vi "main 0.9.0.vi"() -> ()   [LabVIEW 2020]
uses:
  subvi/Newport ESP301/Newport ESP301.lvlib
  subvi/sp_manip.llb/sp_manip_lib.lvlib
  subvi/sp_manip.llb/tcp_gateway.lvlib
  subvi/PHOIBOS/DEFINITIONS/DEF_dev_type.ctl
  subvi/PHOIBOS/DEFINITIONS/DEF_dev_state.ctl
  <vilib>/Utility/file.llb/Write Delimited Spreadsheet (DBL).vi
panel:
  in  "BasePath":path=path "C:/Users/femtolab_admin/Desktop"
  in  "cam_liveavg":bool caption="live average"
  out "G2":dbl[](graph)=[263.145, 1605.73, 2749.3099999999995, 2478.555, 1442.25, 1948.3050000000003, 3089.7200000000003, 2536.98, 1326.19, 1765.79, 1232.225, 654.385, 1490.405, 2145.9949999999994, 2745.5350000000003, 2855.805, 2377.34, 3038.8550000000005, 2930.365, 1581.4399999999998, 1915.805, 2285.69, 1454.7, 796.3300000000002, 1536.01, 2295.5749999999994, 2779.0199999999995, 3696.9249999999997, 2846.545, 1289.3599999999997, 1847.72, 1825.405, 803.2200000000001, 899.645, 662.7249999999999, 467.48, 1104.215, 1475.7500000000002, 1531.1799999999996, 1721.645, 2162.135, 2133.0849999999996, 1255.03, 851.9999999999999, 1367.655, 1933.275, 1143.7749999999999, 741.21, 1149.32, 1642.1000000000001, 1020.995, 530.395, 1069.84, 1391.8100000000002, 1042.03, 1818.6999999999998, 4069.855, 5797.8550000000005, 5827.435, 5055.504999999999, 2832.8900000000003, 1841.045, 2277.75, 1826.1050000000002, 1200.9950000000001, 1153.9649999999997, 1637.5700000000002, 1942.64, 2197.6200000000003, 2863.3550000000005, 3618.209999999999, 3665.4650000000006, 2446.0150000000003, 1297.435, 1719.3950000000002, 2087.6949999999997, 1830.3849999999998, 2194.1750000000006, 2078.385, 1316.6150000000002, 1545.65, 2258.02, 2764.9700000000003, 3237.4200000000005, 1775.6750000000002, 414.32499999999993, 416.3499999999999, 394.96999999999997, 916.545, 1994.625, 3344.8700000000003, 3847.5449999999996, 2925.8199999999997, 2678.08, 2296.67, 1098.0200000000002, 1790.3249999999998, 3163.6549999999997, 3836.945, 3560.370000000001, 2904.32, 2978.2800000000007, 2652.4350000000004, 1855.06, 1771.505, 2235.425, 2266.66, 1323.0649999999998, 1657.0400000000004, 2715.995, 2765.325, 3528.2700000000004, 3528.8050000000003, 2683.3199999999997, 2324.45, 3198.8550000000005, 3244.14, 2267.045, 2132.2949999999996, 2030.79, 907.7950000000001, 1260.255, 1373.4299999999998, 1413.51, 1800.5400000000004, 1761.2450000000003, 1803.33, 2071.47, 2702.28, 3012.6950000000006, 3130.8699999999994, 3128.955, 3589.63, 2744.915000000001, 2048.795, 1583.935, 1144.4499999999998, 1851.075, 1980.545, 1512.4350000000002, 581.935, 731.1850000000001, 621.78, 164.225, 0.0, 0.0, 0.0, 0.0, 0.0, 0.0, 0.0, 0.0, 0.0, 0.0, 0.0, 0.0, 0.0, 124.49000000000001, 496.75, 551.67, 103.64, 0.0, 0.0, 0.0, 0.0, 54.11, 80.15, 0.0, 0.0, 0.0, 0.0, 0.0, 0.0, 0.0, 0.0, 0.0, 0.0, 0.0, 0.0, 0.0, 51.42, 410.03499999999997, 580.33, 174.89999999999998, 0.0, 0.0, 0.0, 0.0, 0.0, 0.0, 0.0, 0.0, 0.0, 0.0, 0.0, 0.0, 0.0, 0.0, 0.0, 0.0, 0.0, 0.0, 0.0, 0.0, 0.0, 0.0, 0.0, 0.0, 0.0, 0.0, 0.0, 0.0, 0.0, 0.0, 0.0, 0.0, 0.0, 0.0, 0.0, 0.0, 0.0, 0.0, 0.0, 0.0, 0.0, 490.6700000000001, 1051.7849999999999, 758.91, 53.42, 0.0, 0.0, 0.0, 60.32, 125.305, 0.0, 0.0, 121.69999999999999, 0.0, 0.0, 0.0, 184.825, 263.615, 0.0, 0.0, 0.0, 0.0, 0.0, 389.45000000000005, 1030.345, 1047.415, 81.37, 0.0, 0.0, 0.0, 301.08, 452.075, 74.22, 0.0, 0.0, 0.0, 0.0, 0.0, 0.0, 0.0, 0.0, 139.67000000000002, 572.5749999999999, 971.985, 771.0349999999999, 693.04, 79.35499999999999, 0.0, 0.0, 0.0, 0.0, 0.0, 0.0, 0.0, 0.0, 0.0, 0.0, 0.0, 0.0, 0.0, 0.0, 0.0, 0.0, 0.0, 0.0, 0.0, 0.0, 0.0, 0.0, 0.0, 0.0, 0.0, 0.0, 0.0, 0.0, 0.0, 0.0, 0.0, 0.0, 0.0, 0.0, 0.0, 0.0, 0.0, 0.0, 0.0, 0.0, 0.0, 0.0, 0.0, 0.0, 0.0, 0.0, 0.0, 0.0, 0.0, 0.0, 0.0, 0.0, 0.0, 0.0, 0.0, 0.0, 0.0, 0.0, 0.0, 0.0, 0.0, 0.0, 0.0, 0.0, 0.0, 0.0, 0.0, 0.0, 0.0, 0.0, 0.0, 0.0, 0.0]
  out "cam_fps":dbl=19.771956531604918 caption="FPS" format="%.1g"
  out "sideimg":dbl[][](graph)
  in  "RunNumber":u16=3
  out "sum":dbl=307111.85500000004 format="%#.2g"
  out "max":dbl=632.85
  out "mainimg":dbl[][](graph)
  out "ESP_con?":bool=TRUE caption="ESP301"
  out "phoib_con?":bool caption="PHOIBOS"
  out "manip_con?":bool caption="manipulator"
  out "cam_con?":bool caption="camera"
  in  "main_close":bool
  in  "Tab Control":T1(tab)
  in  "manip_deltas":dbl[](array[numeric])=[0.0, 0.0, 0.0, 0.0, 10.0, 0.0] caption="delta" format="%#.5g"
  in  "aq.mode":enum32{"Radio Selection 1", "Radio Selection 2"}(radio)=enum."Radio Selection 2"
  out "snap_prog":dbl(slide)=1.0 scale=0.0..1.0
  in  "upper threshold":i32=15000
  in  "dark avg":i32=200
  in  "averages":i32=20 caption="N"
  in  "ESP_delta":dbl caption="relative [mm]"
  in  "ESP_-":bool
  in  "ESP_+":bool
  in  "ESP_go":bool
  in  "ESP_dest_t":dbl caption="[fs]"
  in  "ESP_dest":dbl=33.3075 caption="[mm]"
  in  "ESP_set_t0":bool
  in  "phoib_I_6s":dbl=3200.0
  in  "phoib_I_5s":dbl=1450.0
  in  "phoib_I_4s":dbl=4.558
  in  "phoib_I_3s":dbl=-7.0
  in  "phoib_I_2s":dbl=35.0
  in  "phoib_I_1s":dbl=21.9
  in  "phoib_standby":bool
  in  "phoib_set":bool
  out "phoib_I_6":dbl=3200.0 caption="Screen Voltage"
  out "phoib_I_5":dbl=1450.0 caption="Detctor Voltage"
  out "phoib_I_4":dbl=4.558 caption="Work Function"
  out "phoib_I_3":dbl=-7.0 caption="Coil Current"
  out "phoib_I_2":dbl=35.0 caption="Pass Energy"
  out "phoib_I_1":dbl=21.9 caption="Kinetic Energy"
  out "Saved Positions":string[][](table)=[["ertwertwert", "-2.299945", "-2.030214", "38.900024", "50.000762", "0.000887", "-97.998082"], ["uztgugt", "-14.999451", "-13.638894", "442.380066", "13.998380", "-1.893758", "-76.305838"], ["asdf", "-14.999451", "-13.638894", "442.380066", "13.998380", "-1.893758", "-76.305838"], ["test3", "-14.999451", "-13.638894", "441.380066", "13.998380", "-1.893758", "-76.305838"]]
  in  "Save Pos":bool
  in  "Load":bool
  in  "Delete":bool
  in  "ManipRel +":bool
  in  "ManipRel -":bool
  in  "Move Abs":bool
  in  "stop manip":bool
  in  "dest":dbl[](array[numeric])=[-2.6172862113166087, -0.009888298846365134, 68.5008544921875, -46.36280498847848, 1.1073518432055398, -218.56360350415366] caption="destination" format="%#.5g"
  out "axis":string[](array[string])=["x", "y", "z", "polar", "tilt", "azimut"]
  out "pos":dbl[](array[numeric])=[-2.6172862113166087, -0.009888298846365134, 68.5008544921875, -46.363686276590336, 11.108982061941884, -218.56360350415366] caption="position" format="%.5f"
  in  "Mode":T2(ring)=enum."WideAngleMode"
  in  "VoltageRange":enum16{"3.5kV", "1.5kV", "400V", "100V", "10V"}(ring)=enum."400V"
  out "ESP_pos":dbl=31.8299 caption="Position"
  out "ESP_delay":dbl=1000.0251574040519 caption="Delay"
  out "ESP_t0":dbl=31.68 caption="Time Zero @"
  out "phoib_I_7":dbl=-30.0 caption="Conversion Voltage"
  in  "phoib_I_7s":dbl=-30.0
  in  "phoib_I_8s":dbl=0.0039
  in  "phoib_I_9s":dbl=0.0039
  out "phoib_I_8":dbl=0.0039 caption="FD1"
  out "phoib_I_9":dbl=0.0039 caption="FD2"
  in  "gain":bool
  in  "exposure [ms]":u32=50
  in  "binning":u16(ring)=2 items=["X 1", "X 2", "X 4", "X 8"]
  in  "cam_dark?":bool=TRUE caption="subtract dark?"
  in  "cam_dark":bool
  in  "cam_saveimg":bool
  in  "e-size":u8
  in  "lower threshold":i32=50
  in  "count?":bool
  out "ETA":timestamp=timestamp(3543316529.918047 s since 1904-01-01) format="%<%H:%M:%S>T"
  in  "ROI Left":i32=1
  in  "ROI Right":i32=43
  in  "ROI Top":i32=2
  in  "ROI Bottom":i32=30
  out "moving?":bool[](array[boolean])
  in  "delscan_iters":u32=2 caption="iterations"
  out "scangraph":cluster{dbl[], dbl[]}(graph)={[-1000.0, -900.0, -800.0, -700.0, -600.0, -500.0, -400.0, -300.0, -200.0, -100.0, 0.0, 100.0, 200.0, 300.0, 400.0, 500.0, 600.0, 700.0, 800.0, 900.0, 1000.0], [2248493.455, 2199251.9574999977, 2219914.692499999, 2216051.6575000007, 2215958.2724999995, 2212331.0824999996, 2279964.2799999993, 2180338.027499999, 2266636.2549999994, 2285788.987499997, 2245434.3249999993, 2294344.6275000023, 2285044.407499997, 2174516.5600000033, 2247505.4800000004, 2255556.7350000003, 2175127.462499999, 2208174.432500001, 2235161.732500001, 2220116.9325000024, 2249237.3274999997, 0.0, 0.0, 0.0, 0.0, 0.0, 0.0, 0.0, 0.0, 0.0, 0.0, 0.0, 0.0, 0.0, 0.0, 0.0, 0.0, 0.0, 0.0, 0.0, 0.0, 0.0]}
  in  "delscan_abort":bool
  out "delscan_progress":u32(slide)=20 scale=0.0..21.0
  in  "delscan_go":bool
  out "delscan_pos":dbl=31.829896229 caption="current delay [fs]"
  in  "delscan_end":dbl=1000.0 caption="end [fs]"
  in  "delscan_stepsize":dbl=100.0 caption="stepsize [fs]"
  in  "delscan_start":dbl=-1000.0 caption="start [fs]"
  out "iteration":i32=2
  in  "manip_scan_steps":u32=3
  in  "Optimize":bool
  in  "manip_scan_delta":dbl[](array[numeric])=[0.0, 0.0, 0.0, 0.0, 1.0, 0.0] caption="delta" format="%#.5g"
  out "delscan_progress 2":u32(slide)=2 scale=0.0..3.0
  in  "abort":bool
  in  "manip_init":bool
  in  "manip_release":bool
  in  "phoib_init":bool
  in  "phoib_release":bool
  in  "ESP_init":bool
  in  "ESP_release":bool
  in  "ESP301 VISA":refnum<visa-resource-name>="COM8"
  in  "board number":i32
  in  "cam_init":bool
  in  "cam_release":bool
  out "cam_error":errorcluster
  out "phoib_error":errorcluster
  out "state":T3=1 items=["Off"=-1, "Standby"=0, "On"=1]
  in  "ESP Axis":i32=1 min=1 max=3
  out "error out":errorcluster
  out "error out 2":errorcluster={"status"=TRUE, "code"=1, "source"="TCP Write in sp_manip_lib.lvlib:sp_manip_disconnect.vi->main 0.9.vi"}
  # "camera"
  # "analyzer"
  # "manipulator"
  # "aquisition"
  # "delay stage"
  # "Position"
  # "Destination"
  # "X\nY\nZ\npolar\ntilt\nazimut"
  # "camera"
  # "phoibos"
  # "ESP301"
  # "manipulator"
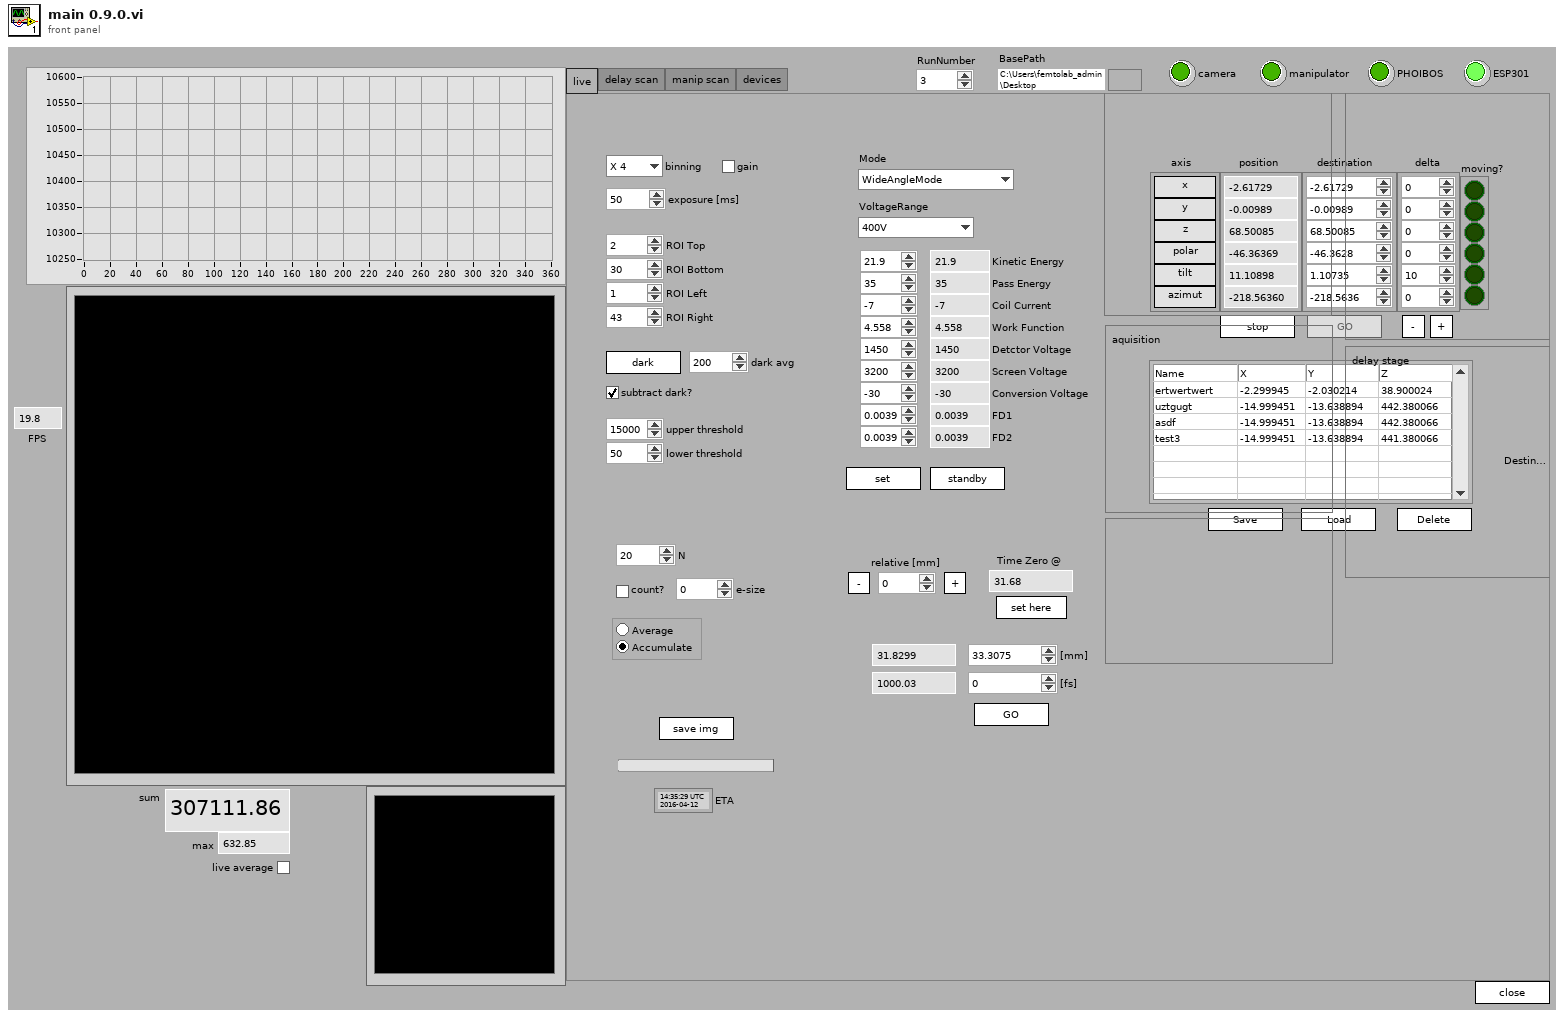
[diagram p1: front panel]
types:
  T1 = enum32{"live", "delay scan", "manip scan", "devices"}
  T2 = enum16{"HighMagnification", "MediumMagnification", "LowMagnification", "HighAngularDispersion", "MediumAngularDispersion", "LowAngularDispersion", "WideAngleMode", "LargeArea", "MediumArea", "SmallArea", "HighMagnification2", "SmallArea2", "ImagingMode"}
  T3 = typedef "DEF_dev_state.ctl" = i32
  T4 = typedef "LVCursorListTypeDef.ctl" = cluster{"Name":string, "Color":u32, "Style":u8, "Point Style":u8, "Name Visible":bool, "Allow Drag":bool, "Cursor Mode":u32, "Plot":i32, "Index":i32, "Position":cluster{"X":dbl, "Y":dbl}, "X Scale":u32, "Y Scale":u32, "Watch Plots":i32[], "Watch All Plots":bool, "Plot Area":i32, "Label Offset":cluster{"X":dbl, "Y":dbl}}[]
  T5 = cluster{"Name":string, "Color":u32, "Style":u8, "Point Style":u8, "Name Visible":bool, "Allow Drag":bool, "Cursor Mode":u32, "Plot":i32, "Index":i32, "Position":cluster{"X":dbl, "Y":dbl}, "X Scale":u32, "Y Scale":u32, "Watch Plots":i32[], "Watch All Plots":bool, "Plot Area":i32, "Label Offset":cluster{"X":dbl, "Y":dbl}}
  T6 = cluster{"Camera type":u32, "Operating mode\nHP & QE / HS & DiCam Pro ":u32, "Frame trigger \n(High Performance and QE only)":u16, "Sequence trigger":u16, "Low Light\n(QE only)":bool, "Gain":bool, "Horzontal\nbinning":u16, "Vertical\nbinning ":u16, "ROI Left":i32, "ROI Right":i32, "ROI Top":i32, "ROI Bottom":i32}
  T7 = cluster{"Axis_Name":string, "Axis_Type":string, "Axis_Position":dbl, "continous":bool, "moving":bool}[]
  T8 = typedef "DEF_dev_type.ctl" = enum32{"devA (analyzer)", "devD (detector)"}
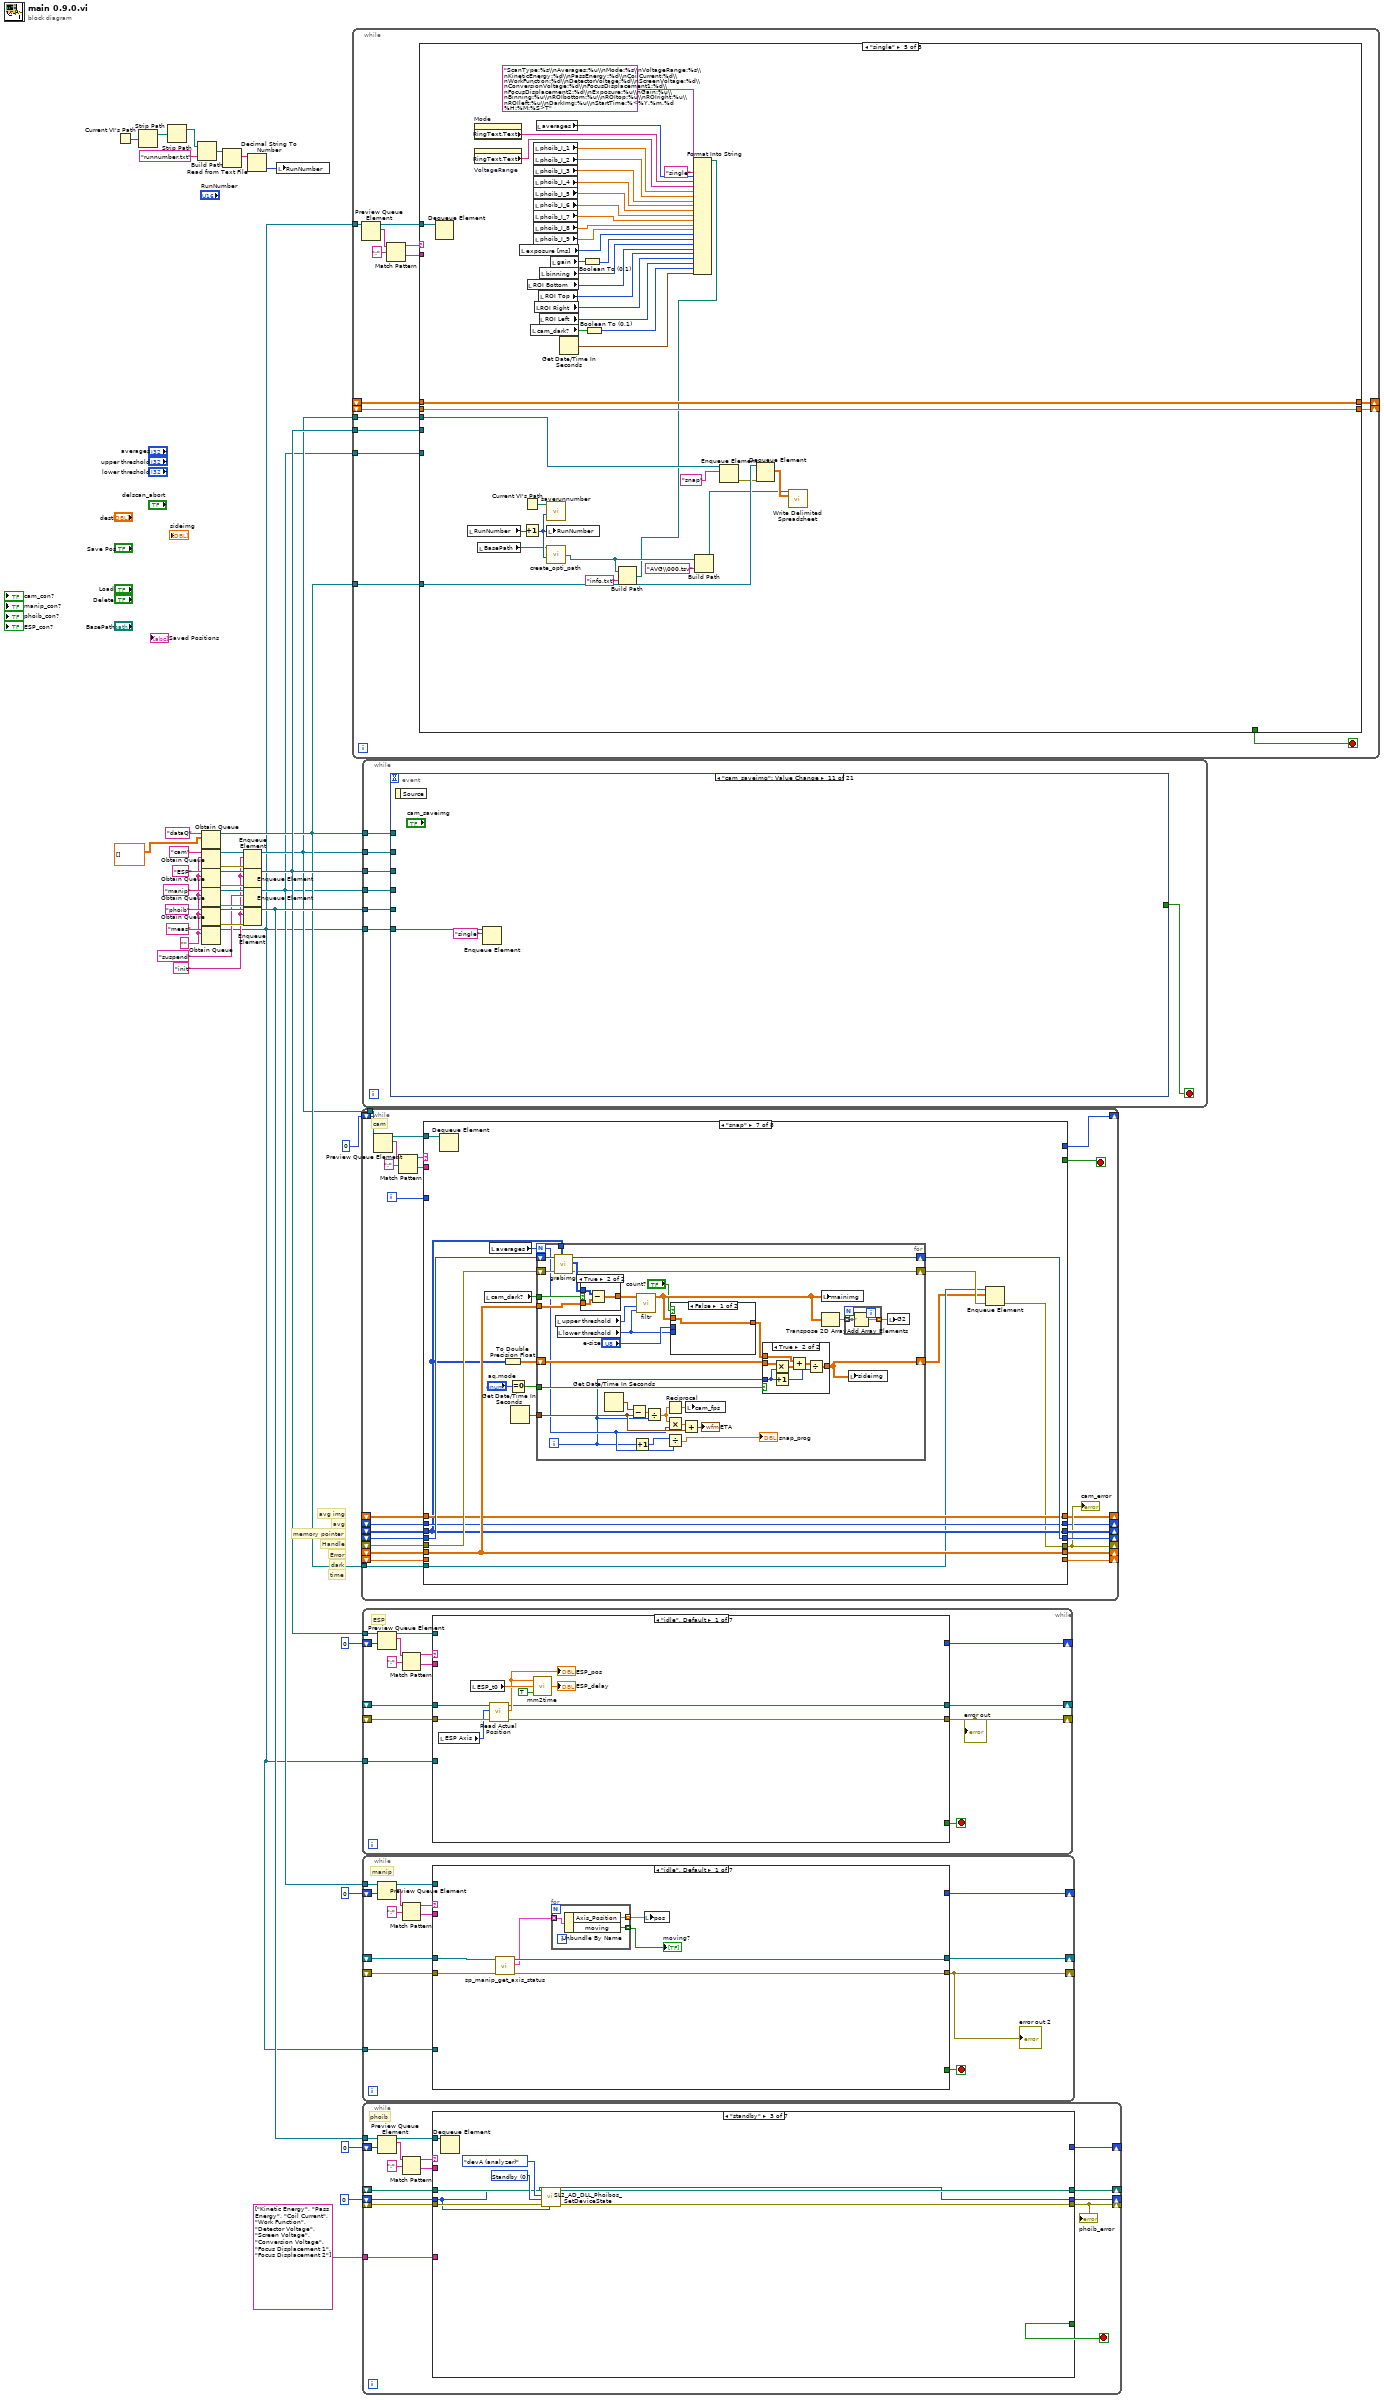
[diagram p0: block diagram]
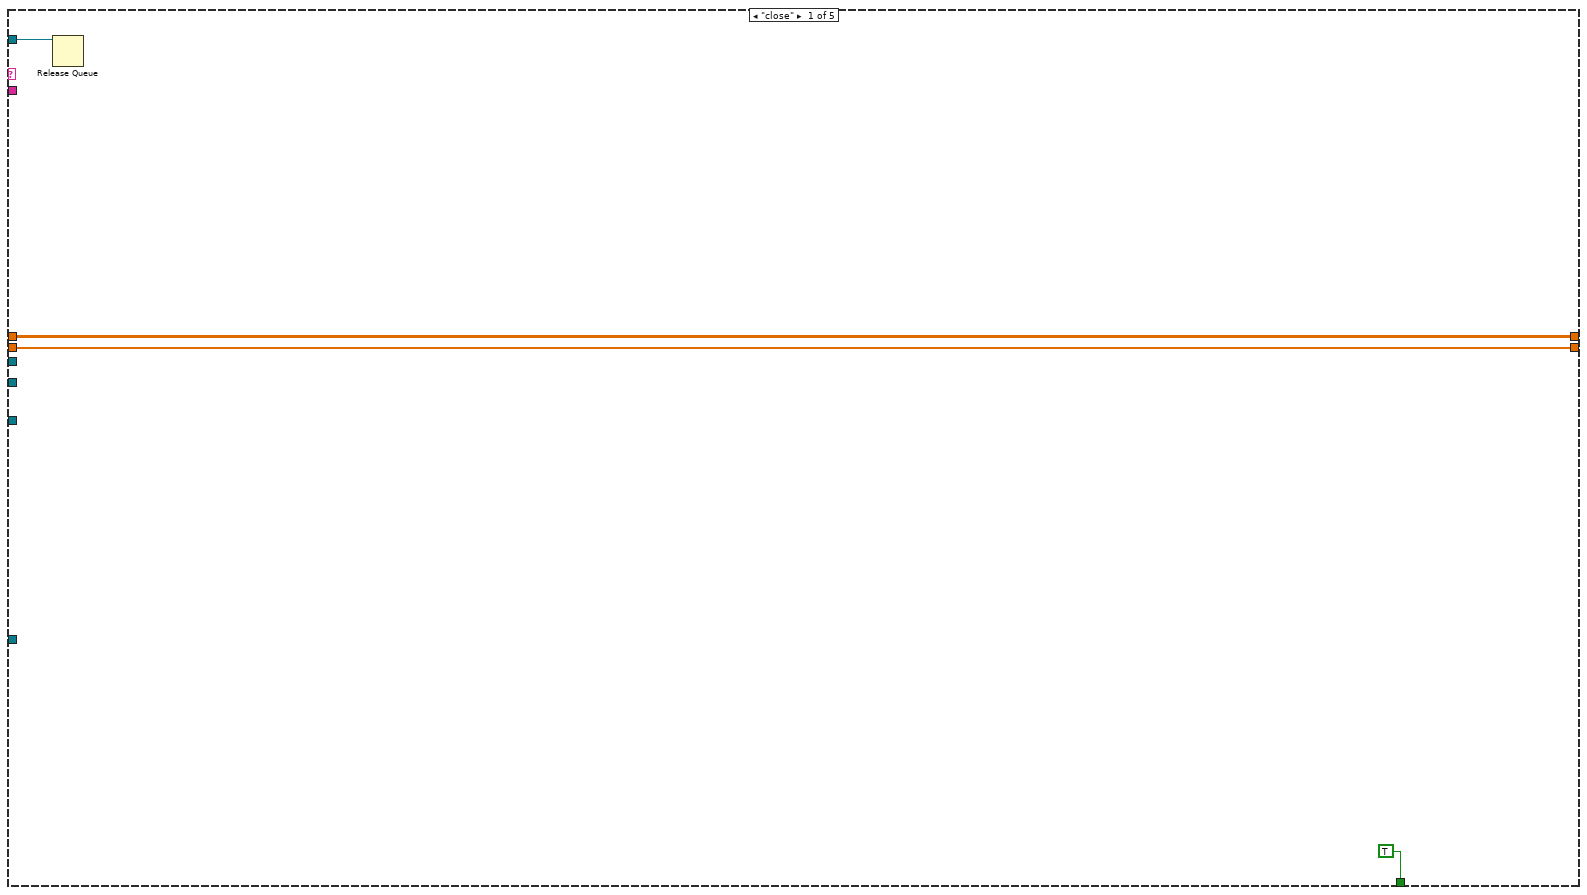
[diagram p2: hidden frame]
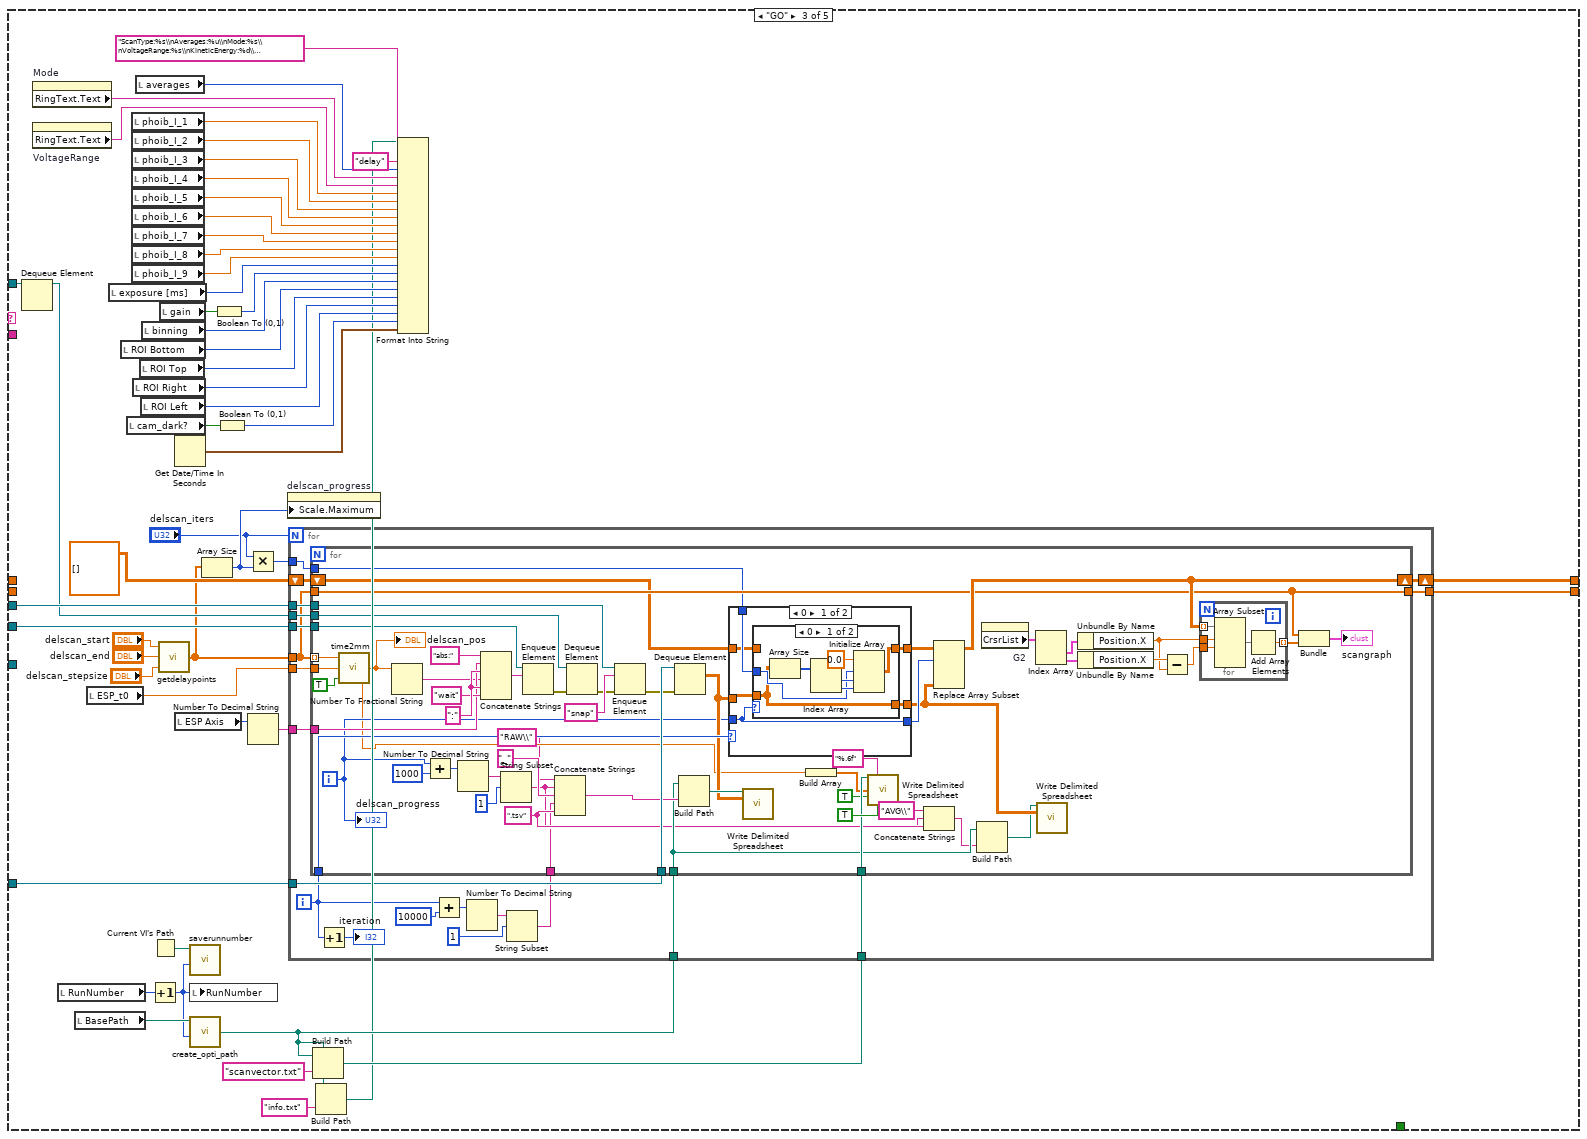
[diagram p4: hidden frame]
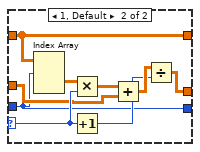
[diagram p6: hidden frame]
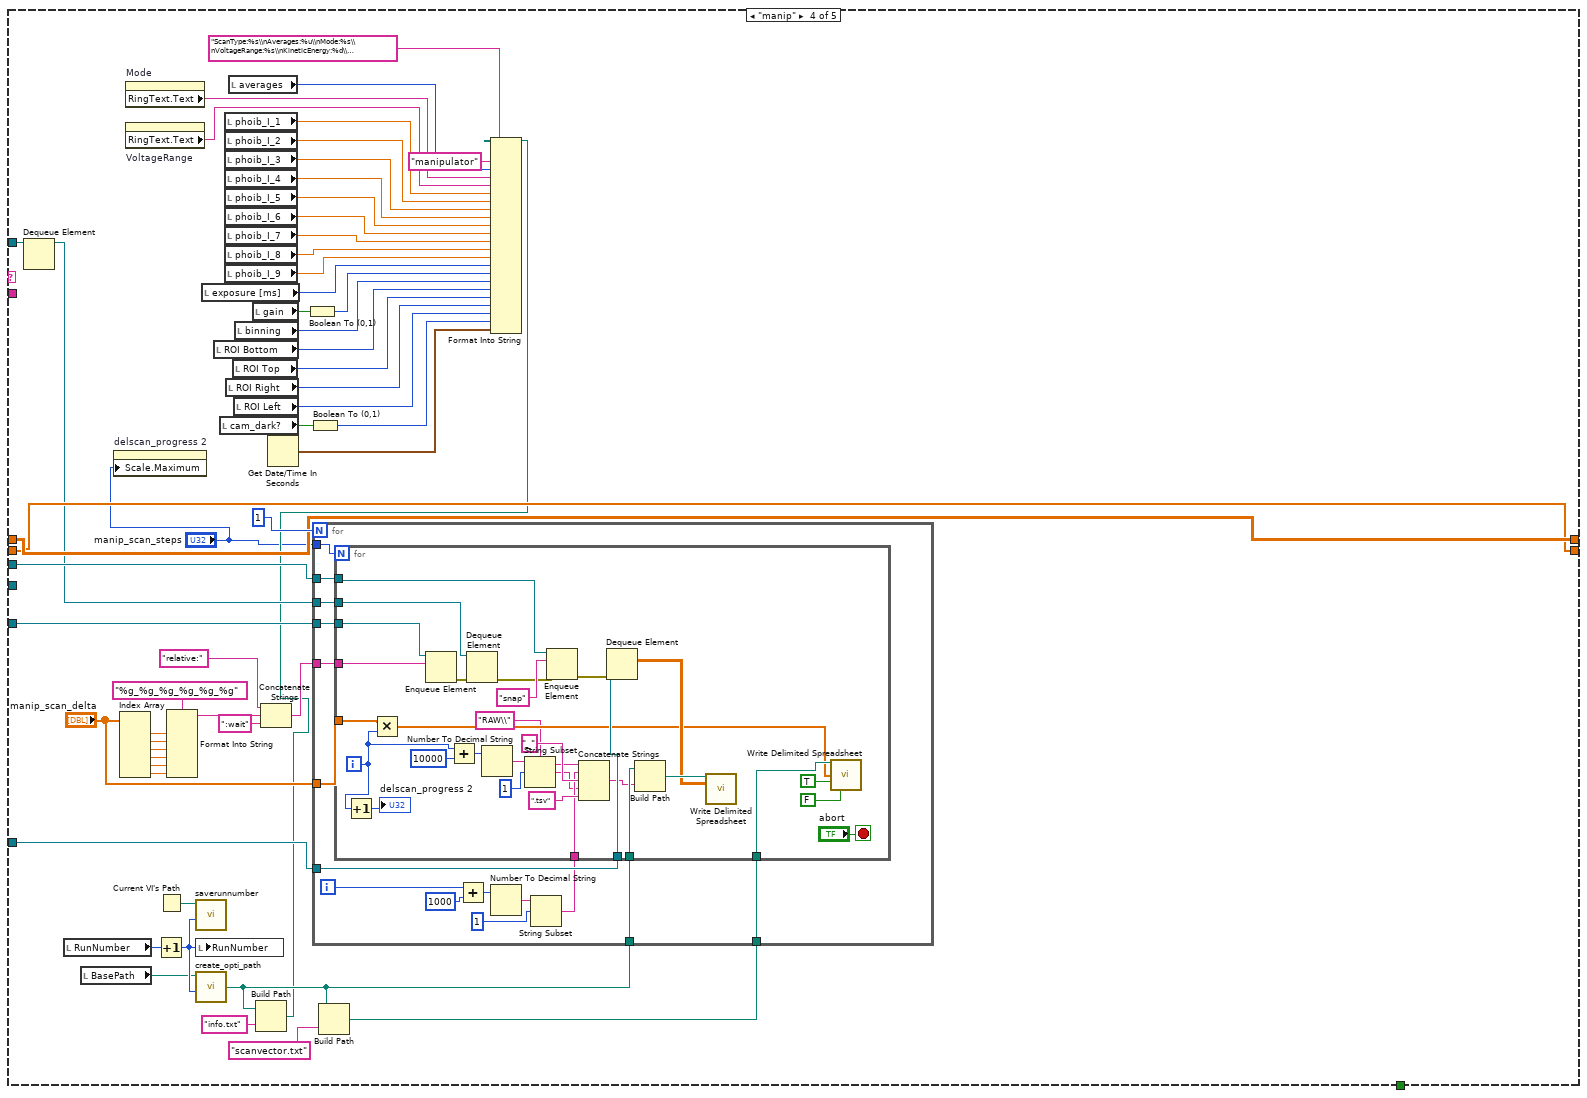
[diagram p7: hidden frame]
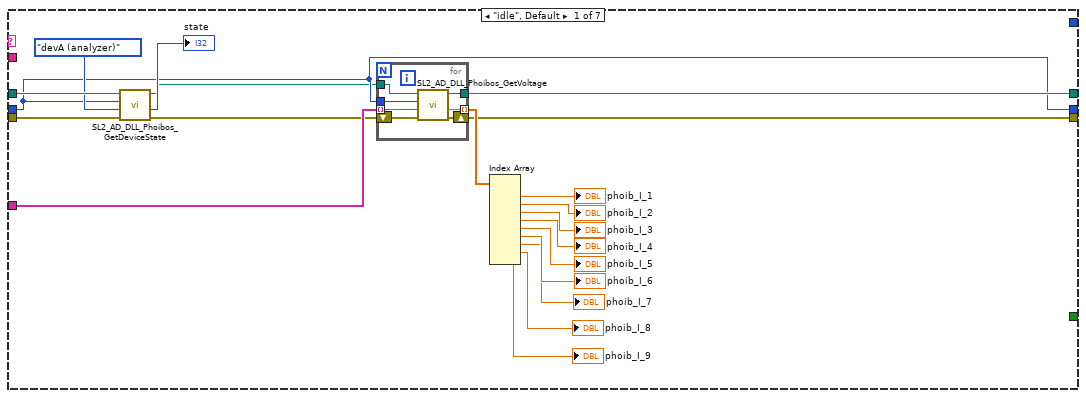
[diagram p8: hidden frame]
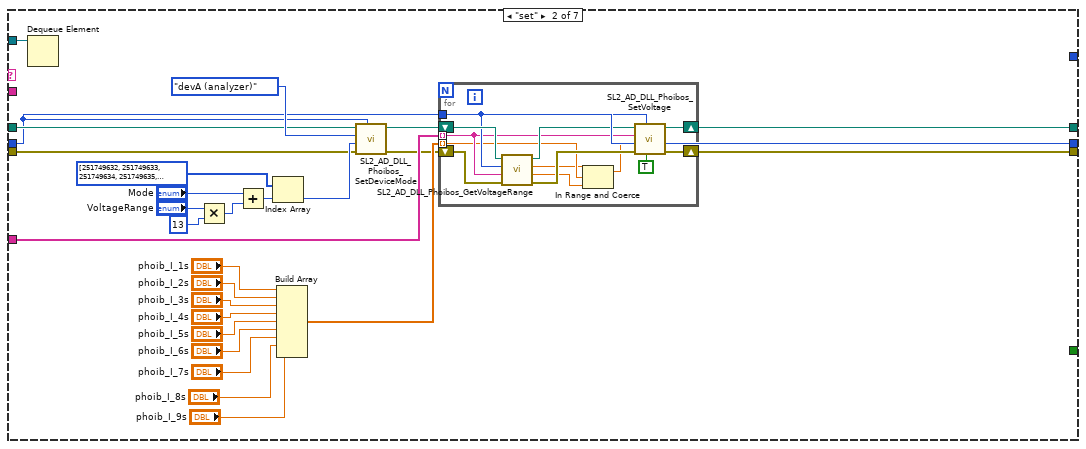
[diagram p9: hidden frame]
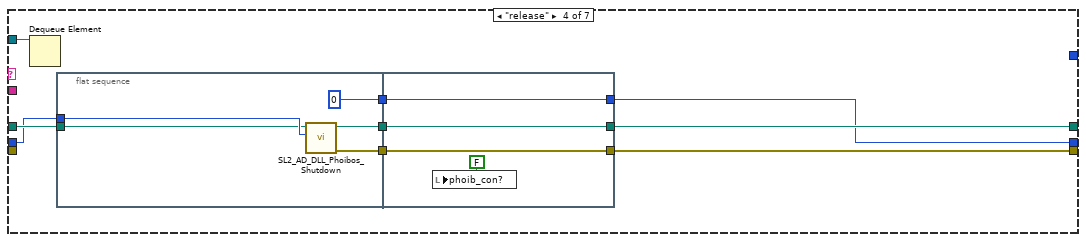
[diagram p10: hidden frame]
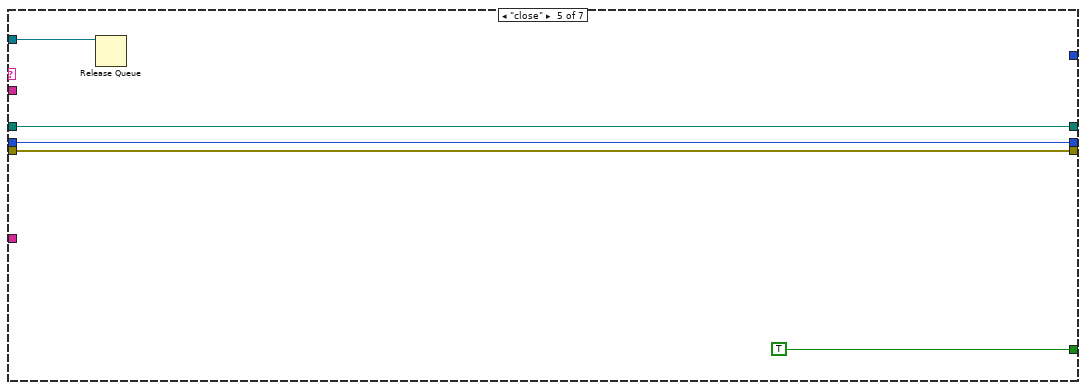
[diagram p11: hidden frame]
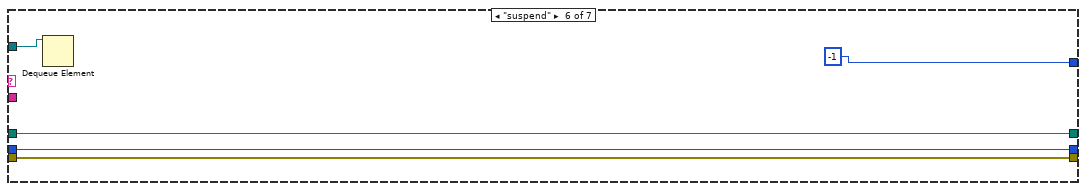
[diagram p12: hidden frame]
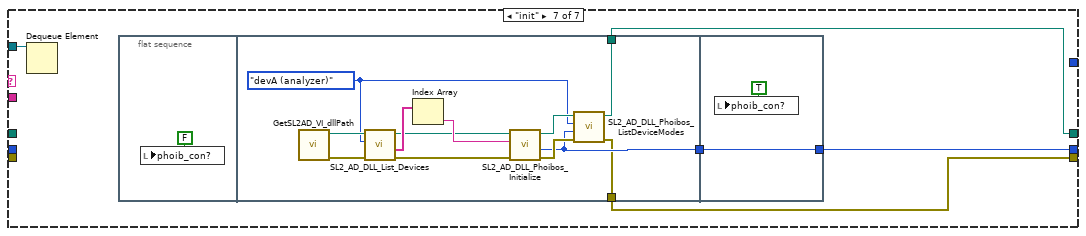
[diagram p13: hidden frame]
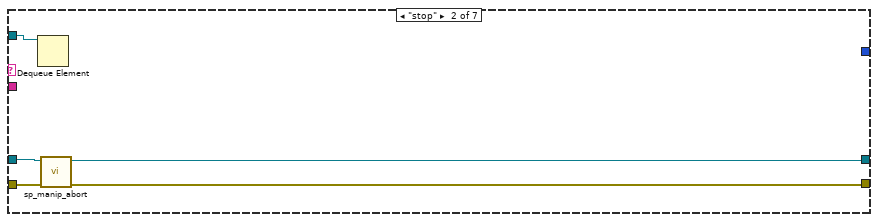
[diagram p14: hidden frame]
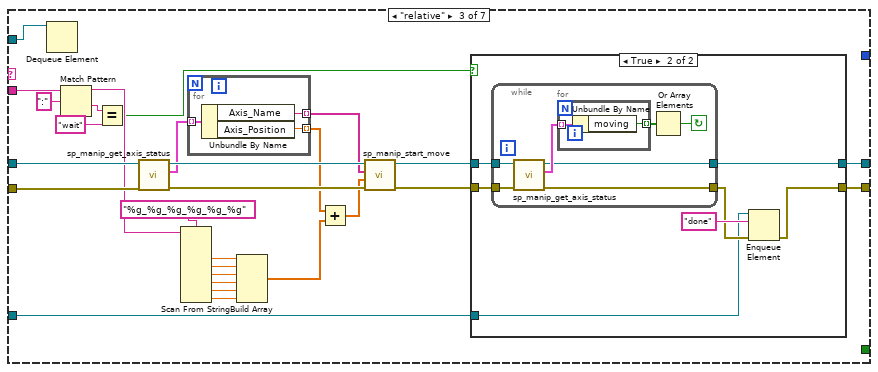
[diagram p15: hidden frame]
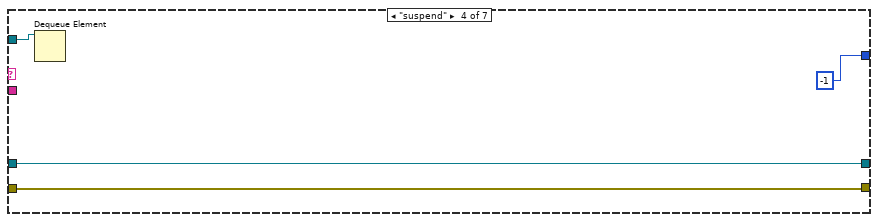
[diagram p17: hidden frame]
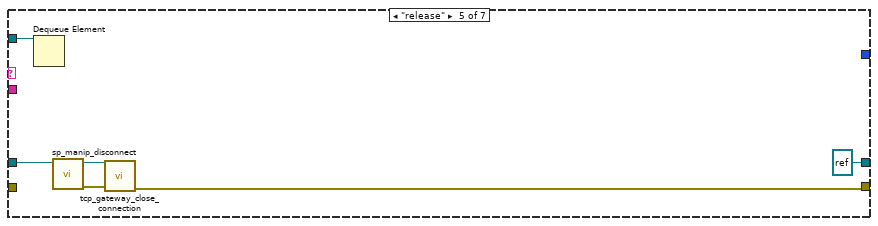
[diagram p18: hidden frame]
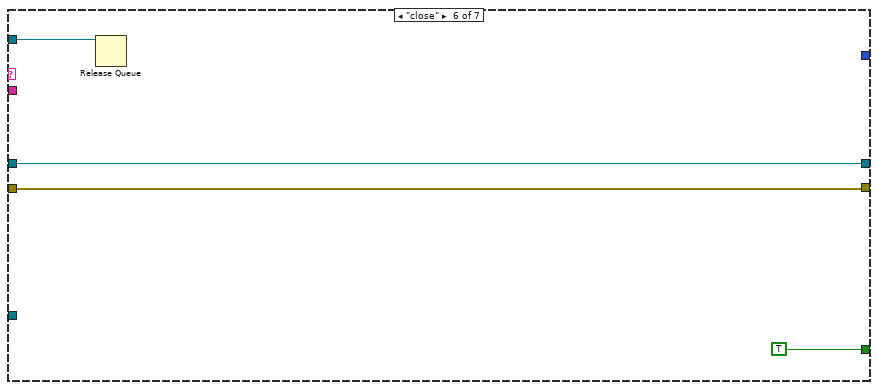
[diagram p19: hidden frame]
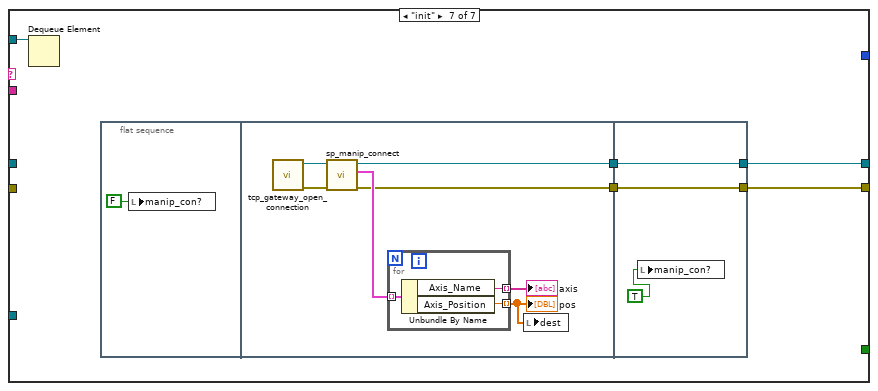
[diagram p20: hidden frame]
diagram:
  w14 = "init" ("name (unnamed)")
  w16 = "" ("name (unnamed)")
  # "avg img"
  # "avg"
  # "time"
  # "dark"
  # "Error"
  # "Handle"
  # "memory pointer"
  n1 = Current VI's Path() -> (path=w4:path)
  n2 = Strip Path(path=w4) -> (stripped path=w8:path)  [unwired: 1 out]
  n3 = Strip Path(path=w8) -> (stripped path=w9:path)  [unwired: 1 out]
  n4 = Build Path(base path=w9, name or relative path="runnumber.txt") -> (appended path=w6:path)
  n5 = Obtain Queue(name (unnamed)="dataQ", element data type=dbl[][] []) -> (queue out=w11:refnum<queue>)  [unwired: 3 in, 2 out]
  n6 = Obtain Queue(name (unnamed)="cam", element data type=w16) -> (queue out=w36:refnum<queue>, error out=w35:errorcluster)  [unwired: 3 in, 1 out]
  n7 = Obtain Queue(name (unnamed)="ESP", element data type=w16) -> (queue out=w33:refnum<queue>, error out=w34:errorcluster)  [unwired: 3 in, 1 out]
  n8 = Obtain Queue(name (unnamed)="manip", element data type=w16) -> (queue out=w30:refnum<queue>, error out=w29:errorcluster)  [unwired: 3 in, 1 out]
  n9 = Obtain Queue(name (unnamed)="phoib", element data type=w16) -> (queue out=w27:refnum<queue>, error out=w28:errorcluster)  [unwired: 3 in, 1 out]
  n10 = Obtain Queue(name (unnamed)="meas", element data type=w16) -> (queue out=w2:refnum<queue>)  [unwired: 3 in, 2 out]
  n11 = Read from Text File(file (use dialog)=w6) -> (text=w7:string)  [unwired: 3 in, 3 out]
  n12 = Enqueue Element(queue=w36, element=w14, error in (no error)=w35) -> (queue out=w10:refnum<queue>)  [unwired: 1 in, 2 out]
  n13 = Enqueue Element(queue=w33, element=w14, error in (no error)=w34) -> (queue out=w13:refnum<queue>)  [unwired: 1 in, 2 out]
  n14 = Enqueue Element(queue=w30, element="suspend" ("name (unnamed)"), error in (no error)=w29) -> (queue out=w3:refnum<queue>)  [unwired: 1 in, 2 out]
  n15 = Enqueue Element(queue=w27, element=w14, error in (no error)=w28) -> (queue out=w24:refnum<queue>)  [unwired: 1 in, 2 out]
  n16 = Decimal String To Number(string=w7) -> (number=w1:i32)  [unwired: 2 in, 1 out]
  n17 = local write "RunNumber"(w1) -> ()
  n18 = while {
    tunnel: w11 -> [w52]
    tunnel: w13 -> [w51]
    tunnel: w10 -> [w50]
    shift-right: [w47] -> _
    shift-left: _ -> [w49]
    shift-right: [w46] -> _
    shift-left: _ -> [w48]
    tunnel: w2 -> [w43]
    tunnel: w3 -> [w38]
    stop <- w39 stop-if-true
    n19 = Preview Queue Element(queue=w43) -> (queue out=w40:refnum<queue>, element=w45:string)  [unwired: 2 in, 2 out]
    n20 = Match Pattern(string=w45, regular expression=":") -> (before substring=w42:string, after substring=w41:string)  [unwired: 1 in, 2 out]
    n21 = case shown="\"single\"" w42 {
      tunnel: w52 -> [_ _ w110 w252 w355]
      tunnel: w51 -> [_ _ w109 _ _]
      tunnel: w50 -> [_ _ w108 w251 w357]
      tunnel: w49 -> [w54 w58 _ w248 w354]
      tunnel: w48 -> [w53 w57 _ w247 w353]
      tunnel: [w54 w58 w107 w248 w354] -> w47
      tunnel: [w53 w57 w95 w247 w353] -> w46
      tunnel: w41 -> [_ _ _ _ _]
      tunnel: w40 -> [w56 _ w97 w246 w356]
      tunnel: [TRUE _ _ _ _] -> w39
      tunnel: w38 -> [_ _ _ w250 _]
      frame "close" {
        n22 = Release Queue(queue=w56) -> ()  [unwired: 2 in, 3 out]
      }
      frame "idle", Default {
      }
      frame "GO" {
        n23 = Dequeue Element(queue=w97) -> (queue out=w96:refnum<queue>)  [unwired: 2 in, 3 out]
        n24 = property on="Mode" class="Enum (strict)"() -> ("RingText.Text"=w84:string)  [unwired: 2 in, 2 out]
        n25 = property on="VoltageRange" class="Enum (strict)"() -> ("RingText.Text"=w83:string)  [unwired: 2 in, 2 out]
        n26 = local read "RunNumber"() -> (w105:u16)
        n27 = local read "BasePath"() -> (w104:path)
        n28 = local read "ESP_t0"() -> (w100:dbl)
        n29 = local read "exposure [ms]"() -> (w73:u32)
        n30 = local read "ROI Bottom"() -> (w70:i32)
        n31 = local read "cam_dark?"() -> (w87:bool)
        n32 = local read "phoib_I_1"() -> (w82:dbl)
        n33 = local read "phoib_I_2"() -> (w81:dbl)
        n34 = local read "phoib_I_3"() -> (w80:dbl)
        n35 = local read "phoib_I_4"() -> (w79:dbl)
        n36 = local read "phoib_I_5"() -> (w78:dbl)
        n37 = local read "phoib_I_6"() -> (w77:dbl)
        n38 = local read "phoib_I_7"() -> (w76:dbl)
        n39 = local read "phoib_I_8"() -> (w75:dbl)
        n40 = local read "phoib_I_9"() -> (w74:dbl)
        n41 = local read "ROI Right"() -> (w68:i32)
        n42 = local read "averages"() -> (w85:i32)
        n43 = local read "ROI Top"() -> (w69:i32)
        n44 = local read "ROI Left"() -> (w67:i32)
        n45 = local read "binning"() -> (w71:u16)
        n46 = Increment(x=w105) -> (x+1=w103:u16)
        n47 = Current VI's Path() -> (path=w106:path)
        n48 = call "getdelaypoints.vi"("delscan_stepsize"="delscan_stepsize", "delscan_end"="delscan_end", "delscan_start"="delscan_start") -> ("delaypoints"=w90:dbl[])
        n49 = local read "gain"() -> (w88:bool)
        n50 = Get Date/Time In Seconds() -> (seconds since 1Jan1904=w65:timestamp)
        n51 = local read "ESP Axis"() -> (w102:i32)
        n52 = call "saverunnumber.vi"("RunNumber"=w103, "VI path"=w106) -> ()  [unwired: 10 in]
        n53 = local write "RunNumber"(w103) -> ()
        n54 = call "create_opti_path.vi"("RunNumber"=w103, "base path"=w104) -> ("Path"=w63:path)  [unwired: 2 in]
        n55 = Array Size(array=w90) -> (size(s)=w94:i32)
        n56 = Boolean To (0,1)(Boolean=w88) -> (0, 1=w72:i16)
        n57 = Boolean To (0,1)(Boolean=w87) -> (0, 1=w66:i16)
        n58 = Multiply(x="delscan_iters", y=w94) -> (x*y=w92:u32)
        n59 = Number To Decimal String(number=w102) -> (decimal integer string=w99:string)  [unwired: 1 in]
        n60 = property on="delscan_progress" class="Slide (strict)"("Scale.Maximum"=w94) -> ()  [unwired: 2 in, 2 out]
        n61 = Build Path(base path=w63, name or relative path="scanvector.txt") -> (appended path=w89:path)
        n62 = for {
          N: "delscan_iters" -> [_]
          tunnel: w90 -> [w114]
          tunnel: w100 -> [w130]
          tunnel: w99 -> [w129]
          tunnel: w109 -> [w127]
          tunnel: w110 -> [w126]
          tunnel: w96 -> [w125]
          tunnel: w108 -> [w124]
          tunnel: w63 -> [w123]
          shift-right: [w121] -> w107
          shift-left: dbl[][][] [] -> [w122]
          tunnel: [w113] -> w95
          tunnel: w92 -> [w112]
          tunnel: w89 -> [w111]
          i -> [w116]
          n63 = Increment(x=w116) -> (x+1=→"iteration":i32)
          n64 = Add(x=w116, y=10000) -> (x+y=w119:i32)
          n65 = Number To Decimal String(number=w119) -> (decimal integer string=w118:string)  [unwired: 1 in]
          n66 = String Subset(string=w118, offset (0)=1) -> (substring=w115:string)  [unwired: 1 in]
          n67 = for {
            tunnel: w114 -> [w180] mode=indexing
            tunnel: w130 -> [w163]
            tunnel: w129 -> [w179]
            tunnel: w127 -> [w178]
            tunnel: w126 -> [w168]
            tunnel: w125 -> [w177]
            tunnel: w124 -> [w176]
            tunnel: w123 -> [w138]
            shift-right: [w154] -> w121
            shift-left: w122 -> [w147]
            tunnel: w116 -> [w162]
            tunnel: w115 -> [w131]
            tunnel: w114 -> [w148]
            tunnel: [w148] -> w113
            tunnel: w112 -> [w146]
            tunnel: w111 -> [w144]
            i -> [w158]
            w135 = ".tsv" ("string")
            w182 = ":" ("string")
            n68 = call "time2mm.vi"("fs[1]/ps[0]"=TRUE, "Offset (mm)"=w163, "time"=w180) -> ("position (mm)"=w141:dbl)
            "delscan_pos" <- w141
            n69 = Number To Fractional String(number=w141) -> (F-format string=w164:string)  [unwired: 3 in]
            n70 = Add(x=w158, y=1000) -> (x+y=w174:i32)
            n71 = Number To Decimal String(number=w174) -> (decimal integer string=w173:string)  [unwired: 1 in]
            n72 = Concatenate Strings("abs:" ("string"), w179, w182, w164, w182, "wait" ("string")) -> (w186:string)
            n73 = String Subset(string=w173, offset (0)=1) -> (substring=w132:string)  [unwired: 1 in]
            n74 = Enqueue Element(queue=w178, element=w186) -> (error out=w183:errorcluster)  [unwired: 2 in, 2 out]
            n75 = Concatenate Strings("RAW\\" ("string"), w132, "_" ("string"), w131, w135) -> (w165:string)
            n76 = Dequeue Element(queue=w177, error in (no error)=w183) -> (error out=w169:errorcluster)  [unwired: 1 in, 3 out]
            n77 = Enqueue Element(queue=w176, element="snap", error in (no error)=w169) -> (error out=w167:errorcluster)  [unwired: 1 in, 2 out]
            n78 = Dequeue Element(queue=w168, error in (no error)=w167) -> (element=w161:dbl[][])  [unwired: 1 in, 3 out]
            n79 = Build Path(base path=w138, name or relative path=w165) -> (appended path=w166:path)
            n80 = case shown="0" w162 {
              selector: w162 -> [_ w214]
              tunnel: w147 -> [w194 w207]
              tunnel: w158 -> [w192 w208]
              tunnel: w161 -> [w197 w210]
              tunnel: [w193 w207] -> w160
              tunnel: [w195 w211] -> w139
              tunnel: [w192 w208] -> w159
              tunnel: w146 -> [w196 _]
              frame 0 {
                n81 = case shown="0" w192 {
                  tunnel: w197 -> [w199 w206]
                  tunnel: w196 -> [w200 _]
                  tunnel: [w199 w206] -> w195
                  tunnel: w194 -> [_ w205]
                  tunnel: [w198 w205] -> w193
                  frame 0 {
                    n82 = Array Size(array=w199) -> (size(s)=w203:i32[])
                    n83 = Index Array(array=w203) -> (element #1=w202:i32, element #2=w201:i32)  [unwired: 2 in]
                    n84 = Initialize Array(0.0 ("element"), w200, w202, w201) -> (w198:dbl[][][])
                  }
                  frame 1, Default {
                  }
                }
              }
              frame 1, Default {
                n85 = Index Array(array=w207, index (dim 0)=w208) -> (element=w215:dbl[][])  [unwired: 2 in]
                n86 = Multiply(x=w215, y=w214) -> (x*y=w209:dbl[][])
                n87 = Increment(x=w214) -> (x+1=w212:i32)
                n88 = Add(x=w209, y=w210) -> (x+y=w213:dbl[][])
                n89 = Divide(x=w213, y=w212) -> (x/y=w211:dbl[][])
              }
            }
            n90 = call-poly <vilib>:"Write Delimited Spreadsheet.vi"("file path (dialog if empty)"=w166, "2D data"=w161) -> ()  [unwired: 12 in, 2 out]
            n91 = Build Array(w141) -> (w142:dbl[])
            n92 = call-poly <vilib>:"Write Delimited Spreadsheet.vi"("file path (dialog if empty)"=w144, "format (%.3f)"="%.6f", "1D data"=w142, "append to file? (new file:F)"=TRUE ("append to file? (F)"), "transpose? (no:F)"=TRUE ("transpose? (F)")) -> ()  [unwired: 9 in, 2 out]
            n93 = Concatenate Strings("AVG\\" ("string"), w132, w135) -> (w137:string)
            n94 = Replace Array Subset(array=w160, new element=w139, index (dim 0)=w159) -> (w154:dbl[][][])  [unwired: 2 in]
            n95 = Build Path(base path=w138, name or relative path=w137) -> (appended path=w134:path)
            n96 = property on="G2" class="WFGraph (strict)"() -> ("CrsrList"=w157:T4)  [unwired: 2 in, 2 out]
            n97 = Index Array(array=w157) -> (element #1=w156:T5, element #2=w155:T5)  [unwired: 2 in]
            n98 = call-poly <vilib>:"Write Delimited Spreadsheet.vi"("file path (dialog if empty)"=w134, "2D data"=w139) -> ()  [unwired: 12 in, 2 out]
            n99 = Unbundle By Name(w156) -> ("Position.X"=w152:dbl)
            n100 = Unbundle By Name(w155) -> ("Position.X"=w153:dbl)
            n101 = Subtract(x=w153, y=w152) -> (x-y=w151:dbl)
            n102 = for {
              tunnel: w154 -> [w191] mode=indexing
              tunnel: w152 -> [w190]
              tunnel: w151 -> [w189]
              tunnel: [w187] -> w150 mode=indexing
              n103 = Array Subset(array=w191, index (row)=w190, length (row)=w189) -> (w188:dbl[][])  [unwired: 2 in]
              n104 = Add Array Elements(numeric array=w188) -> (sum=w187:dbl)
            }
            n105 = Bundle("delaypoints"=w148, w150) -> (→"scangraph":cluster{"delaypoints":dbl[], dbl[]})  [unwired: 1 in]
            "delscan_progress" <- w158
          }
        }
        n106 = Build Path(base path=w63, name or relative path="info.txt") -> (appended path=w62:path)
        n107 = Format Into String(format string="ScanType:%s\\nAverages:%u\\nMode:%s\\nVoltageRange:%s\\nKineticEnergy:%d\\nPassEnergy:%d\\nCoilCurrent:%d\\nWorkFunction:%d\\nDetectorVoltage:%d\\nScreenVoltage:%d\\nConversionVoltage:%d\\nFocusDisplacement1:%d\\nFocusDisplacement2:%d\\nExposure:%u\\nGain:%u\\nBinning:%u\\nROIbottom:%u\\nROItop:%u\\nROIright:%u\\nROIleft:%u\\nDarkImg:%u\\nStartTime:%<%Y.%m.%d %H:%M:%S>T", initial string=w62, "delay" ("input 1"), w85, w84, w83, w82, w81, w80, w79, w78, w77, w76, w75, w74, w73, w72, w71, w70, w69, w68, w67, w66, w65) -> ()  [unwired: 1 in, 2 out]
      }
      frame "manip" {
        n108 = Dequeue Element(queue=w246) -> (queue out=w245:refnum<queue>)  [unwired: 2 in, 3 out]
        n109 = local read "RunNumber"() -> (w254:u16)
        n110 = local read "BasePath"() -> (w255:path)
        n111 = property on="delscan_progress 2" class="Slide (strict)"("Scale.Maximum"="manip_scan_steps") -> ()  [unwired: 2 in, 2 out]
        n112 = Index Array(array="manip_scan_delta") -> (element #1=w267:dbl, element #2=w266:dbl, element #3=w265:dbl, element #4=w264:dbl, element #5=w263:dbl, element #6=w262:dbl)  [unwired: 6 in]
        n113 = property on="Mode" class="Enum (strict)"() -> ("RingText.Text"=w240:string)  [unwired: 2 in, 2 out]
        n114 = property on="VoltageRange" class="Enum (strict)"() -> ("RingText.Text"=w239:string)  [unwired: 2 in, 2 out]
        n115 = Increment(x=w254) -> (x+1=w256:u16)
        n116 = Current VI's Path() -> (path=w253:path)
        n117 = Format Into String(format string="%g_%g_%g_%g_%g_%g", w267, w266, w265, w264, w263, w262) -> (resulting string=w260:string)  [unwired: 2 in, 1 out]
        n118 = call "saverunnumber.vi"("RunNumber"=w256, "VI path"=w253) -> ()  [unwired: 10 in]
        n119 = local write "RunNumber"(w256) -> ()
        n120 = call "create_opti_path.vi"("RunNumber"=w256, "base path"=w255) -> ("Path"=w219:path)  [unwired: 2 in]
        n121 = local read "exposure [ms]"() -> (w229:u32)
        n122 = local read "ROI Bottom"() -> (w226:i32)
        n123 = local read "cam_dark?"() -> (w243:bool)
        n124 = local read "phoib_I_1"() -> (w238:dbl)
        n125 = local read "phoib_I_2"() -> (w237:dbl)
        n126 = local read "phoib_I_3"() -> (w236:dbl)
        n127 = local read "phoib_I_4"() -> (w235:dbl)
        n128 = local read "phoib_I_5"() -> (w234:dbl)
        n129 = local read "phoib_I_6"() -> (w233:dbl)
        n130 = local read "phoib_I_7"() -> (w232:dbl)
        n131 = local read "phoib_I_8"() -> (w231:dbl)
        n132 = local read "phoib_I_9"() -> (w230:dbl)
        n133 = local read "ROI Right"() -> (w224:i32)
        n134 = local read "averages"() -> (w241:i32)
        n135 = local read "ROI Top"() -> (w225:i32)
        n136 = local read "ROI Left"() -> (w223:i32)
        n137 = local read "binning"() -> (w227:u16)
        n138 = local read "gain"() -> (w244:bool)
        n139 = Build Path(base path=w219, name or relative path="info.txt") -> (appended path=w218:path)
        n140 = Concatenate Strings("relative:" ("string"), w260, ":wait" ("string")) -> (w269:string)
        n141 = Get Date/Time In Seconds() -> (seconds since 1Jan1904=w221:timestamp)
        n142 = Boolean To (0,1)(Boolean=w244) -> (0, 1=w228:i16)
        n143 = Boolean To (0,1)(Boolean=w243) -> (0, 1=w222:i16)
        n144 = Build Path(base path=w219, name or relative path="scanvector.txt") -> (appended path=w270:path)
        n145 = for {
          N: 1 -> [_]
          tunnel: w252 -> [w285]
          tunnel: w219 -> [w284]
          tunnel: w270 -> [w277]
          tunnel: "manip_scan_steps" -> [w276]
          tunnel: w269 -> [w275]
          tunnel: w250 -> [w274]
          tunnel: w245 -> [w273]
          tunnel: w251 -> [w272]
          tunnel: "manip_scan_delta" -> [w271]
          i -> [w279]
          n146 = Add(x=w279, y=1000) -> (x+y=w282:i32)
          n147 = Number To Decimal String(number=w282) -> (decimal integer string=w281:string)  [unwired: 1 in]
          n148 = String Subset(string=w281, offset (0)=1) -> (substring=w278:string)  [unwired: 1 in]
          n149 = for {
            N: w276 -> [_]
            tunnel: w285 -> [w308]
            tunnel: w284 -> [w305]
            tunnel: w278 -> [w299]
            tunnel: w277 -> [w301]
            tunnel: w275 -> [w296]
            tunnel: w274 -> [w295]
            tunnel: w273 -> [w294]
            tunnel: w272 -> [w293]
            tunnel: w271 -> [w291]
            i -> [w286]
            stop <- "abort" stop-if-true
            n150 = Increment(x=w286) -> (x+1=→"delscan_progress 2":i32)
            n151 = Multiply(x=w291, y=w286) -> (x*y=w290:dbl[])
            n152 = Enqueue Element(queue=w295, element=w296) -> (error out=w297:errorcluster)  [unwired: 2 in, 2 out]
            n153 = Add(x=w286, y=10000) -> (x+y=w314:i32)
            n154 = Dequeue Element(queue=w294, error in (no error)=w297) -> (error out=w292:errorcluster)  [unwired: 1 in, 3 out]
            n155 = Number To Decimal String(number=w314) -> (decimal integer string=w313:string)  [unwired: 1 in]
            n156 = String Subset(string=w313, offset (0)=1) -> (substring=w298:string)  [unwired: 1 in]
            n157 = Enqueue Element(queue=w293, element="snap", error in (no error)=w292) -> (error out=w307:errorcluster)  [unwired: 1 in, 2 out]
            n158 = Concatenate Strings("RAW\\" ("string"), w299, "_" ("string"), w298, ".tsv" ("string")) -> (w304:string)
            n159 = Dequeue Element(queue=w308, error in (no error)=w307) -> (element=w303:dbl[][])  [unwired: 1 in, 3 out]
            n160 = Build Path(base path=w305, name or relative path=w304) -> (appended path=w306:path)
            n161 = call-poly <vilib>:"Write Delimited Spreadsheet.vi"("file path (dialog if empty)"=w306, "2D data"=w303) -> ()  [unwired: 12 in, 2 out]
            n162 = call-poly <vilib>:"Write Delimited Spreadsheet.vi"("file path (dialog if empty)"=w301, "1D data"=w290, "append to file? (new file:F)"=TRUE ("append to file? (F)"), "transpose? (no:F)"=FALSE ("transpose? (F)")) -> ()  [unwired: 10 in, 2 out]
          }
        }
        n163 = Format Into String(format string="ScanType:%s\\nAverages:%u\\nMode:%s\\nVoltageRange:%s\\nKineticEnergy:%d\\nPassEnergy:%d\\nCoilCurrent:%d\\nWorkFunction:%d\\nDetectorVoltage:%d\\nScreenVoltage:%d\\nConversionVoltage:%d\\nFocusDisplacement1:%d\\nFocusDisplacement2:%d\\nExposure:%u\\nGain:%u\\nBinning:%u\\nROIbottom:%u\\nROItop:%u\\nROIright:%u\\nROIleft:%u\\nDarkImg:%u\\nStartTime:%<%Y.%m.%d %H:%M:%S>T", initial string=w218, "manipulator" ("input 1"), w241, w240, w239, w238, w237, w236, w235, w234, w233, w232, w231, w230, w229, w228, w227, w226, w225, w224, w223, w222, w221) -> ()  [unwired: 1 in, 2 out]
      }
      frame "single" {
        n164 = Dequeue Element(queue=w356) -> ()  [unwired: 2 in, 4 out]
        n165 = local read "RunNumber"() -> (w347:u16)
        n166 = property on="Mode" class="Enum (strict)"() -> ("RingText.Text"=w341:string)  [unwired: 2 in, 2 out]
        n167 = property on="VoltageRange" class="Enum (strict)"() -> ("RingText.Text"=w340:string)  [unwired: 2 in, 2 out]
        n168 = local read "BasePath"() -> (w348:path)
        n169 = local read "exposure [ms]"() -> (w330:u32)
        n170 = Increment(x=w347) -> (x+1=w349:u16)
        n171 = Current VI's Path() -> (path=w346:path)
        n172 = local read "ROI Bottom"() -> (w327:i32)
        n173 = local read "cam_dark?"() -> (w344:bool)
        n174 = local read "phoib_I_1"() -> (w339:dbl)
        n175 = local read "phoib_I_2"() -> (w338:dbl)
        n176 = local read "phoib_I_3"() -> (w337:dbl)
        n177 = local read "phoib_I_4"() -> (w336:dbl)
        n178 = local read "phoib_I_5"() -> (w335:dbl)
        n179 = local read "phoib_I_6"() -> (w334:dbl)
        n180 = local read "phoib_I_7"() -> (w333:dbl)
        n181 = local read "phoib_I_8"() -> (w332:dbl)
        n182 = local read "phoib_I_9"() -> (w331:dbl)
        n183 = local read "ROI Right"() -> (w325:i32)
        n184 = local read "averages"() -> (w342:i32)
        n185 = local read "ROI Top"() -> (w326:i32)
        n186 = local read "ROI Left"() -> (w324:i32)
        n187 = local read "binning"() -> (w328:u16)
        n188 = call "saverunnumber.vi"("RunNumber"=w349, "VI path"=w346) -> ()  [unwired: 10 in]
        n189 = local write "RunNumber"(w349) -> ()
        n190 = call "create_opti_path.vi"("RunNumber"=w349, "base path"=w348) -> ("Path"=w319:path)  [unwired: 2 in]
        n191 = local read "gain"() -> (w345:bool)
        n192 = Get Date/Time In Seconds() -> (seconds since 1Jan1904=w322:timestamp)
        n193 = Boolean To (0,1)(Boolean=w345) -> (0, 1=w329:i16)
        n194 = Boolean To (0,1)(Boolean=w344) -> (0, 1=w323:i16)
        n195 = Build Path(base path=w319, name or relative path="info.txt") -> (appended path=w317:path)
        n196 = Format Into String(format string="ScanType:%s\\nAverages:%u\\nMode:%s\\nVoltageRange:%s\\nKineticEnergy:%d\\nPassEnergy:%d\\nCoilCurrent:%d\\nWorkFunction:%d\\nDetectorVoltage:%d\\nScreenVoltage:%d\\nConversionVoltage:%d\\nFocusDisplacement1:%d\\nFocusDisplacement2:%d\\nExposure:%u\\nGain:%u\\nBinning:%u\\nROIbottom:%u\\nROItop:%u\\nROIright:%u\\nROIleft:%u\\nDarkImg:%u\\nStartTime:%<%Y.%m.%d %H:%M:%S>T", initial string=w317, "single" ("input 1"), w342, w341, w340, w339, w338, w337, w336, w335, w334, w333, w332, w331, w330, w329, w328, w327, w326, w325, w324, w323, w322) -> ()  [unwired: 1 in, 2 out]
        n197 = Build Path(base path=w319, name or relative path="AVG\\000.tsv") -> (appended path=w320:path)
        n198 = Enqueue Element(queue=w357, element="snap" ("string")) -> (error out=w351:errorcluster)  [unwired: 2 in, 2 out]
        n199 = Dequeue Element(queue=w355, error in (no error)=w351) -> (element=w350:dbl[][])  [unwired: 1 in, 3 out]
        n200 = call-poly <vilib>:"Write Delimited Spreadsheet.vi"("file path (dialog if empty)"=w320, "2D data"=w350) -> ()  [unwired: 12 in, 2 out]
      }
    }
  }
  n201 = while {
    tunnel: w10 -> [w382]
    shift-right: [w376] -> _
    shift-left: _ -> [w375]
    shift-right: [w374] -> _
    shift-left: _ -> [w372]
    shift-right: [w373] -> _
    shift-left: _ -> [w371]
    shift-right: [w368] -> _
    shift-left: 0 -> [w369]
    shift-right: [w367] -> _
    shift-left: _ -> [w366]
    shift-right: [w365] -> _
    shift-left: _ -> [w364]
    tunnel: w11 -> [w363]
    shift-right: [w362] -> _
    shift-left: _ -> [w361]
    shift-right: [w359] -> _
    shift-left: _ -> [w358]
    i -> [w360]
    stop <- w370 stop-if-true
    # "cam"
    n202 = Preview Queue Element(queue=w382, timeout in ms (-1)=w369) -> (queue out=w381:refnum<queue>, element=w380:string)  [unwired: 1 in, 2 out]
    n203 = Match Pattern(string=w380, regular expression=":") -> (before substring=w377:string, after substring=w378:string)  [unwired: 1 in, 2 out]
    n204 = case shown="\"snap\"" w377 {
      tunnel: w381 -> [w392 w422 w450 w462 _ w519 w547 w611]
      tunnel: w378 -> [_ _ _ _ _ _ _ _]
      tunnel: [w386 w408 w449 w460 w467 w516 w536 w609] -> w376
      tunnel: w375 -> [_ _ w449 w460 w467 w516 w536 w609]
      tunnel: [w391 w423 u64 0 ("Hout") w459 w477 w517 w542 w608] -> w374
      tunnel: [w393 w424 w446 w458 w478 w518 w530 w607] -> w373
      tunnel: w372 -> [_ w426 w448 w459 w480 w521 w544 w608]
      tunnel: w371 -> [_ w425 _ w458 w479 w520 w543 w607]
      tunnel: [_ _ _ TRUE _ _ _ _] -> w370
      tunnel: [_ _ _ _ _ _ _ -1] -> w368
      tunnel: [w385 w409 _ _ w488 _ _ _] -> w367
      tunnel: w366 -> [w385 w409 _ _ w487 _ _ _]
      tunnel: [w386 w411 w444 w457 w483 w510 w545 w606] -> w365
      tunnel: w364 -> [_ w411 w444 w457 w483 _ w545 w606]
      tunnel: w363 -> [_ _ _ _ _ _ w534 _]
      tunnel: [w383 w406 w443 w455 w464 w507 w539 w605] -> w362
      tunnel: w361 -> [w383 w406 w443 w455 w471 w507 w539 w605]
      tunnel: w360 -> [_ _ _ _ w470 _ _ _]
      tunnel: [w384 w407 w442 w456 w469 w506 w538 w604] -> w359
      tunnel: w358 -> [w384 w407 w442 w456 w468 w506 w538 w604]
      frame "init" {
        w386 = u16[][] []
        n205 = flat-sequence {
          tunnel: [w395] -> w390
          tunnel: [w396] -> w389
          tunnel: [w404] -> w391
          tunnel: [w405] -> w393
          tunnel: w390 -> [w405]
          tunnel: w389 -> [w404]
          frame #0 {
            n206 = local write "cam_con?"(FALSE ("cam_con?")) -> ()
          }
          frame #1 {
            n207 = call "SCInitBoard.vi"("boardnr"="board number") -> ("Hout"=w399:u32, "error out"=w400:errorcluster)  [unwired: 1 in, 1 out]
            n208 = call "SCSetupCamera.vi"("Handle"=w399, "error in (no error)"=w400) -> ("Hout"=w401:u64, "error out"=w402:errorcluster)  [unwired: 1 out]
            n209 = call "SCStopCOC.vi"("error in (no error)"=w402, "Stop mode"=0, "Handle"=w401) -> ("error out"=w395:errorcluster, "Hout"=w396:u64)
          }
          frame #2 {
            n210 = local write "cam_con?"(TRUE ("cam_con?")) -> ()
          }
        }
        n211 = Dequeue Element(queue=w392) -> (queue out=w388:refnum<queue>)  [unwired: 2 in, 3 out]
        n212 = Enqueue Element At Opposite End(queue=w388, element="set") -> ()  [unwired: 2 in, 3 out]
      }
      frame "set" {
        w421 = u32 1 ("Operating mode\nHP & QE / HS & DiCam Pro")
        n213 = Dequeue Element(queue=w422) -> ()  [unwired: 2 in, 4 out]
        n214 = Bundle By Name(cluster=cluster{"Delay":dbl, "Exposure ":dbl} {"Delay"=0.0, "Exposure "=0.0} ("Delay and exposure"), "Exposure"="exposure [ms]") -> (w418:cluster{"Delay":dbl, "Exposure ":dbl})
        n215 = call "SCStopCOC.vi"("error in (no error)"=w425, "Stop mode"=0, "Handle"=w426) -> ("error out"=w441:errorcluster, "Hout"=w440:u64)
        n216 = Bundle By Name(cluster=T6 {"Camera type"=0, "Operating mode\nHP & QE / HS & DiCam Pro "=0, "Frame trigger \n(High Performance and QE only)"=0, "Sequence trigger"=0, "Low Light\n(QE only)"=FALSE, "Gain"=FALSE, "Horzontal\nbinning"=0, "Vertical\nbinning "=0, "ROI Left"=1, "ROI Right"=20, "ROI Top"=1, "ROI Bottom"=15} ("Camera controls"), "Operating mode\nHP & QE / HS & DiCam Pro"=w421, "Horzontal\nbinning"="binning", "Vertical\nbinning"="binning", "ROI Left"="ROI Left", "ROI Right"="ROI Right", "ROI Top"="ROI Top", "ROI Bottom"="ROI Bottom", "Gain"="gain") -> (w436:T6)
        n217 = call "New delay and exposure forma.vi"("Operating mode\nHP & QE / HS & DiCam Pro"=w421, "Delay and exposure"=w418) -> ("Output table"=w437:string)  [unwired: 3 in]
        n218 = call "SCSetCoC.vi"("error in (no error)"=w441, "Delay and exposure table"=w437, "Camera controls"=w436, "Handle"=w440) -> ("error out"=w429:errorcluster, "Hout"=w428:u64)  [unwired: 1 out]
        n219 = call "SCGetImageSize.vi"("Handle"=w428, "error in (no error)"=w429) -> ("Hout"=w427:u64, "error out"=w410:errorcluster, "Horizontal size"=w415:i32, "Vertical size"=w414:i32)  [unwired: 2 out]
        n220 = Greater?(x=w415, y=w414) -> (0:w416:bool)
        n221 = Initialize Array(u16 0 ("dimension size"), w414, w415) -> (w408:u16[][])
        n222 = call "SCRun.vi"("error in (no error)"=w410, "Run mode"=0, "Handle"=w427) -> ("error out"=w424:errorcluster, "Hout"=w423:u64)  [unwired: 1 out]
        n223 = Select(t=w415, s=w416, f=w414) -> (s? t:f=w413:i32)
        n224 = property on="mainimg" class="IntGraph (strict)"("XScale.Maximum"=w413, "YScale.Maximum"=w413) -> ()  [unwired: 2 in, 2 out]
      }
      frame "release" {
        n225 = Dequeue Element(queue=w450) -> ()  [unwired: 2 in, 4 out]
        n226 = flat-sequence {
          tunnel: w448 -> [w452]
          tunnel: [w451] -> w445
          tunnel: [w454] -> w446
          tunnel: w445 -> [w454]
          frame #0 {
            n227 = call "SCCloseBoard.vi"("Handle"=w452) -> ("error out"=w451:errorcluster)  [unwired: 1 in, 2 out]
          }
          frame #1 {
            n228 = local write "cam_con?"(FALSE ("cam_con?")) -> ()
          }
        }
      }
      frame "close" {
        n229 = Release Queue(queue=w462) -> ()  [unwired: 2 in, 3 out]
      }
      frame "idle", Default {
        n230 = call "grabimg.vi"("array in"=w467, "error in"=w479, "Hin"=w480) -> ("error out"=w478:errorcluster, "imgdata"=w476:i32[][], "Hout"=w477:u64)  [unwired: 6 in]
        n231 = local read "upper threshold"() -> (w463:i32)
        n232 = local read "lower threshold"() -> (w474:i32)
        n233 = case shown="False" "cam_dark?" {
          tunnel: w483 -> [_ w505]
          tunnel: [w502 w504] -> w475
          tunnel: w476 -> [w502 w503]
          frame False {
          }
          frame True {
            n234 = Subtract(x=w503, y=w505) -> (x-y=w504:dbl[][])
          }
        }
        n235 = call "filtr.vi"("lower threshold"=w474, "upper threshold"=w463, "input array"=w475) -> ("output array"=w472:dbl[][])  [unwired: 8 in]
        n236 = call <vilib>:"High Resolution Relative Seconds.vi"() -> ("relative seconds"=w488:dbl)
        n237 = Subtract(x=w488, y=w487) -> (x-y=w486:dbl)
        n238 = Reciprocal(x=w486) -> (1/x=→"cam_fps":dbl)
        n239 = case shown="False" "cam_liveavg" {
          tunnel: w472 -> [w491 w497]
          tunnel: [w491 w493] -> w464
          tunnel: w471 -> [_ w499]
          tunnel: w470 -> [w492 w501]
          tunnel: [w492 w500] -> w469
          tunnel: w468 -> [_ w500]
          frame False {
          }
          frame True {
            n240 = Subtract(x=w501, y=w500) -> (x-y=w495:i32)
            n241 = Multiply(x=w499, y=w495) -> (x*y=w498:dbl[][])
            n242 = Increment(x=w495) -> (x+1=w494:i32)
            n243 = Add(x=w498, y=w497) -> (x+y=w496:dbl[][])
            n244 = Divide(x=w496, y=w494) -> (x/y=w493:dbl[][])
          }
        }
        "mainimg" <- w464
        n245 = Array Max & Min(array=w464) -> (max value=→"max":dbl)  [unwired: 3 out]
        n246 = Add Array Elements(numeric array=w464) -> (sum=→"sum":dbl)
        n247 = Transpose 2D Array(2D array=w464) -> (transposed array=w465:dbl[][])
        n248 = for {
          tunnel: w465 -> [w490] mode=indexing
          tunnel: [w489] -> w466 mode=indexing
          n249 = Add Array Elements(numeric array=w490) -> (sum=w489:dbl)
        }
        "G2" <- w466
      }
      frame "dark" {
        n250 = Dequeue Element(queue=w519) -> ()  [unwired: 2 in, 4 out]
        n251 = Array Size(array=w516) -> (size(s)=w515:i32[])
        n252 = Index Array(array=w515) -> (element #1=w514:i32, element #2=w513:i32)  [unwired: 2 in]
        n253 = Initialize Array(0.0 ("element"), w514, w513) -> (w511:dbl[][])
        n254 = for {
          N: "dark avg" -> [_]
          tunnel: w521 -> [w529]
          tunnel: w520 -> [w528]
          tunnel: [w527] -> w518
          tunnel: w516 -> [w526]
          tunnel: [w525] -> w517
          shift-right: [w522] -> w509
          shift-left: w511 -> [w523]
          n255 = call "grabimg.vi"("array in"=w526, "error in"=w528, "Hin"=w529) -> ("error out"=w527:errorcluster, "imgdata"=w524:i32[][], "Hout"=w525:u64)  [unwired: 6 in]
          n256 = Add(x=w524, y=w523) -> (x+y=w522:dbl[][])
        }
        n257 = Divide(x=w509, y="dark avg") -> (x/y=w510:dbl[][])
      }
      frame "snap" {
        n258 = Dequeue Element(queue=w547) -> ()  [unwired: 2 in, 4 out]
        n259 = local read "cam_dark?"() -> (w546:bool)
        n260 = local read "averages"() -> (w541:i32)
        n261 = To Double Precision Float(number=w536) -> (double precision float=w535:dbl[][])
        n262 = Equal To 0?(x="aq.mode") -> (x = 0?=w532:bool)
        n263 = Get Date/Time In Seconds() -> (seconds since 1Jan1904=w537:timestamp)
        n264 = for {
          N: w541 -> [w551]
          shift-right: [w576] -> w542
          shift-left: w544 -> [w578]
          shift-right: [w561] -> w540
          shift-left: w543 -> [w577]
          tunnel: w546 -> [w574]
          tunnel: w545 -> [w573]
          tunnel: w536 -> [w572]
          tunnel: w537 -> [w567]
          tunnel: w532 -> [w553]
          shift-right: [w552] -> w531
          shift-left: w535 -> [w554]
          i -> [w548]
          n265 = call "grabimg.vi"("array in"=w572, "error in"=w577, "Hin"=w578) -> ("error out"=w561:errorcluster, "imgdata"=w575:i32[][], "Hout"=w576:u64)  [unwired: 6 in]
          n266 = local read "upper threshold"() -> (w560:i32)
          n267 = local read "lower threshold"() -> (w556:i32)
          n268 = case shown="True" w574 {
            tunnel: w575 -> [w600 w603]
            tunnel: w573 -> [_ w602]
            tunnel: [w600 w601] -> w571
            frame False {
            }
            frame True {
              n269 = Subtract(x=w603, y=w602) -> (x-y=w601:dbl[][])
            }
          }
          n270 = Get Date/Time In Seconds() -> (seconds since 1Jan1904=w570:timestamp)
          n271 = Subtract(x=w570, y=w567) -> (x-y=w569:dbl)
          n272 = Increment(x=w548) -> (x+1=w549:i32)
          n273 = call "filtr.vi"("lower threshold"=w556, "upper threshold"=w560, "input array"=w571) -> ("output array"=w559:dbl[][])  [unwired: 8 in]
          n274 = Divide(x=w569, y=w548) -> (x/y=w565:dbl)
          n275 = Reciprocal(x=w565) -> (1/x=w564:dbl)
          n276 = Multiply(x=w565, y=w551) -> (x*y=w568:dbl)
          n277 = Divide(x=w549, y=w551) -> (x/y=→"snap_prog":dbl)
          n278 = case shown="False" "count?" {
            tunnel: w559 -> [w589 w591]
            tunnel: "e-size" -> [_ w593]
            tunnel: w556 -> [_ w592]
            tunnel: [w589 w590] -> w555
            frame False {
            }
            frame True {
              n279 = Array Size(array=w591) -> (size(s)=w595:i32[])
              n280 = call "findr.vi"("thresh"=w592, "esize"=w593, "inp array"=w591) -> ("locs"=w594:i32[][])  [unwired: 8 in]
              n281 = Index Array(array=w595) -> (element #1=w597:i32, element #2=w596:i32)  [unwired: 2 in]
              n282 = call "drawe.vi"("Ysize"=w597, "Xsize"=w596, "pos array"=w594) -> ("img out"=w590:i32[][])  [unwired: 8 in]
            }
          }
          n283 = Add(x=w568, y=w567) -> (x+y=→"ETA":timestamp)
          n284 = local write "cam_fps"(w564) -> ()
          n285 = case shown="True" w553 {
            tunnel: w555 -> [w579 w587]
            tunnel: w548 -> [_ w586]
            tunnel: w554 -> [w581 w585]
            tunnel: [w580 w582] -> w552
            frame False {
              n286 = Add(x=w579, y=w581) -> (x+y=w580:dbl[][])
            }
            frame True {
              n287 = Multiply(x=w585, y=w586) -> (x*y=w588:dbl[][])
              n288 = Increment(x=w586) -> (x+1=w583:i32)
              n289 = Add(x=w587, y=w588) -> (x+y=w584:dbl[][])
              n290 = Divide(x=w584, y=w583) -> (x/y=w582:dbl[][])
            }
          }
          n291 = local write "mainimg"(w559) -> ()
          n292 = Transpose 2D Array(2D array=w559) -> (transposed array=w562:dbl[][])
          n293 = for {
            tunnel: w562 -> [w599] mode=indexing
            tunnel: [w598] -> w563 mode=indexing
            n294 = Add Array Elements(numeric array=w599) -> (sum=w598:dbl)
          }
          n295 = local write "sideimg"(w552) -> ()
          n296 = local write "G2"(w563) -> ()
        }
        n297 = Enqueue Element(queue=w534, element=w531, error in (no error)=w540) -> (error out=w530:errorcluster)  [unwired: 1 in, 2 out]
      }
      frame "suspend" {
        n298 = Dequeue Element(queue=w611) -> ()  [unwired: 2 in, 4 out]
      }
    }
    "cam_error" <- w373
  }
  n299 = while {
    tunnel: w10 -> [w617]
    tunnel: w13 -> [w616]
    tunnel: w3 -> [w615]
    tunnel: w24 -> [w614]
    tunnel: w2 -> [w612]
    tunnel: w11 -> [w613]
    stop <- w618 stop-if-true
    n300 = event shown="[10] \"cam_saveimg\": Value Change" {
      selector: _ -> [_ _ _ _ _ _ _ _ _ _ _ _ _ _ _ _ _ _ _ _ _]
      dyn-events: _ -> [_ _ _ _ _ _ _ _ _ _ _ _ _ _ _ _ _ _ _ _ _]
      timeout: _ -> [_ _ _ _ _ _ _ _ _ _ _ _ _ _ _ _ _ _ _ _ _]
      tunnel: [_ TRUE _ _ _ _ _ _ _ _ _ _ _ _ _ _ _ _ _ _ _] -> w618
      tunnel: w617 -> [_ w630 w633 _ _ _ _ _ w659 w661 _ _ _ _ _ _ _ _ _ _ _]
      tunnel: w616 -> [_ w629 _ w637 _ _ _ _ _ _ _ _ _ _ _ _ w692 _ w704 _ _]
      tunnel: w615 -> [_ w628 _ _ w643 _ _ _ _ _ _ _ _ w680 _ w684 _ _ _ _ _]
      tunnel: w614 -> [_ w627 _ _ _ w649 w655 w656 _ _ _ _ _ _ _ _ _ _ _ _ _]
      tunnel: w613 -> [_ w621 _ _ _ _ _ _ _ _ _ _ _ _ _ _ _ _ _ _ _]
      tunnel: w612 -> [_ w620 _ _ _ _ _ _ _ _ w663 w665 _ _ w682 _ _ _ _ _ _]
      event Timeout {
        n301 = event-data() -> ()  [unwired: 1 in, 1 out]
      }
      event "main_close": Value Change {
        w619 = "close" ("element")
        w626 = "release" ("element")
        n302 = event-data() -> ()  [unwired: 1 in, 1 out]
        n303 = Release Queue(queue=w621) -> ()  [unwired: 2 in, 3 out]
        n304 = Enqueue Element(queue=w630, element=w626) -> (queue out=w625:refnum<queue>)  [unwired: 2 in, 2 out]
        n305 = Enqueue Element(queue=w629, element=w626) -> (queue out=w624:refnum<queue>)  [unwired: 2 in, 2 out]
        n306 = Enqueue Element(queue=w628, element=w626) -> (queue out=w623:refnum<queue>)  [unwired: 2 in, 2 out]
        n307 = Enqueue Element(queue=w627, element=w626) -> (queue out=w622:refnum<queue>)  [unwired: 2 in, 2 out]
        n308 = Enqueue Element(queue=w625, element=w619) -> ()  [unwired: 2 in, 3 out]
        n309 = Enqueue Element(queue=w624, element=w619) -> ()  [unwired: 2 in, 3 out]
        n310 = Enqueue Element(queue=w623, element=w619) -> ()  [unwired: 2 in, 3 out]
        n311 = Enqueue Element(queue=w622, element=w619) -> ()  [unwired: 2 in, 3 out]
        n312 = Enqueue Element(queue=w620, element=w619) -> ()  [unwired: 2 in, 3 out]
      }
      event "cam_release", "cam_init": Value Change {
        n313 = event-data() -> ()  [unwired: 1 in, 2 out]
        n314 = Select(t="init" ("name (unnamed)"), s="cam_init", f="release" ("name (unnamed)")) -> (s? t:f=w632:string)
        n315 = Enqueue Element(queue=w633, element=w632) -> ()  [unwired: 2 in, 3 out]
      }
      event "ESP_release", "ESP_init": Value Change {
        n316 = event-data() -> ()  [unwired: 1 in, 2 out]
        n317 = Select(t="init" ("name (unnamed)"), s="ESP_init", f="release" ("name (unnamed)")) -> (s? t:f=w641:string)
        n318 = Enqueue Element(queue=w637, element=w641) -> ()  [unwired: 2 in, 3 out]
      }
      event "manip_init", "manip_release": Value Change {
        n319 = event-data() -> ()  [unwired: 1 in, 2 out]
        n320 = Flush Queue(queue=w643) -> (queue out=w642:refnum<queue>)  [unwired: 1 in, 2 out]
        n321 = Select(t="init" ("name (unnamed)"), s="manip_init", f="release" ("name (unnamed)")) -> (s? t:f=w645:string)
        n322 = Enqueue Element(queue=w642, element=w645) -> ()  [unwired: 2 in, 3 out]
      }
      event "phoib_release", "phoib_init": Value Change {
        n323 = event-data() -> ()  [unwired: 1 in, 2 out]
        n324 = Flush Queue(queue=w649) -> (queue out=w648:refnum<queue>)  [unwired: 1 in, 2 out]
        n325 = Select(t="init" ("name (unnamed)"), s="phoib_init", f="release" ("name (unnamed)")) -> (s? t:f=w651:string)
        n326 = Enqueue Element(queue=w648, element=w651) -> ()  [unwired: 2 in, 3 out]
      }
      event "phoib_standby": Value Change {
        n327 = event-data() -> ()  [unwired: 1 in, 2 out]
        n328 = Enqueue Element(queue=w655, element="standby") -> ()  [unwired: 2 in, 3 out]
      }
      event "phoib_set": Value Change {
        n329 = event-data() -> ()  [unwired: 1 in, 2 out]
        n330 = Enqueue Element(queue=w656, element="set") -> ()  [unwired: 2 in, 3 out]
      }
      event "cam_dark": Value Change {
        n331 = event-data() -> ()  [unwired: 1 in, 2 out]
        n332 = Enqueue Element(queue=w659, element="dark") -> ()  [unwired: 2 in, 3 out]
      }
      event "ROI Left", "ROI Right", "ROI Top", "ROI Bottom", "exposure [ms]", "binning", "gain": Value Change {
        n333 = event-data() -> ()  [unwired: 1 in, 1 out]
        n334 = Enqueue Element(queue=w661, element="set") -> ()  [unwired: 2 in, 3 out]
      }
      event "cam_saveimg": Value Change {
        n335 = event-data() -> ()  [unwired: 1 in, 1 out]
        n336 = Enqueue Element(queue=w663, element="single") -> ()  [unwired: 2 in, 3 out]
      }
      event "delscan_go": Value Change {
        n337 = event-data() -> ()  [unwired: 1 in, 1 out]
        n338 = Enqueue Element(queue=w665, element="GO") -> ()  [unwired: 2 in, 3 out]
      }
      event "Move Abs": Value Change {
        n339 = event-data() -> ()  [unwired: 1 in, 1 out]
      }
      event "ManipRel +", "ManipRel -": Value Change {
        n340 = event-data() -> ()  [unwired: 1 in, 2 out]
        n341 = Negate(x="manip_deltas") -> (-x=w668:dbl[])
        n342 = Select(t="manip_deltas", s="ManipRel +", f=w668) -> (s? t:f=w666:dbl[])
        n343 = Index Array(array=w666) -> (element #1=w672:dbl, element #2=w673:dbl, element #3=w674:dbl, element #4=w675:dbl, element #5=w676:dbl, element #6=w677:dbl)  [unwired: 6 in]
        n344 = Format Into String(format string="%g_%g_%g_%g_%g_%g", w672, w673, w674, w675, w676, w677) -> (resulting string=w679:string)  [unwired: 2 in, 1 out]
        n345 = Concatenate Strings("relative:" ("string"), w679) -> (w670:string)
        n346 = Enqueue Element(queue=w680, element=w670) -> ()  [unwired: 2 in, 3 out]
      }
      event "Optimize": Value Change {
        n347 = event-data() -> ()  [unwired: 1 in, 6 out]
        n348 = Enqueue Element(queue=w682, element="manip") -> ()  [unwired: 2 in, 3 out]
      }
      event "stop manip": Value Change {
        n349 = event-data() -> ()  [unwired: 1 in, 1 out]
        n350 = Enqueue Element(queue=w684, element="stop") -> ()  [unwired: 2 in, 3 out]
      }
      event "ESP_go": Value Change {
        w686 = ":" ("string")
        n351 = event-data() -> ()  [unwired: 1 in, 1 out]
        n352 = local read "ESP Axis"() -> (w685:i32)
        n353 = Number To Decimal String(number=w685) -> (decimal integer string=w688:string)  [unwired: 1 in]
        n354 = Number To Fractional String(number="ESP_dest") -> (F-format string=w687:string)  [unwired: 3 in]
        n355 = Concatenate Strings("abs:" ("string"), w688, w686, w687, w686) -> (w691:string)
        n356 = Enqueue Element(queue=w692, element=w691) -> ()  [unwired: 2 in, 3 out]
      }
      event "ESP_set_t0": Value Change {
        n357 = event-data() -> ()  [unwired: 1 in, 1 out]
        n358 = Current VI's Path() -> (path=w698:path)
        n359 = Strip Path(path=w698) -> (stripped path=w694:path)  [unwired: 1 out]
        n360 = Strip Path(path=w694) -> (stripped path=w693:path)  [unwired: 1 out]
        n361 = local read "ESP_pos"() -> (w696:dbl)
        "ESP_t0" <- w696
        n362 = Number To Fractional String(number=w696) -> (F-format string=w695:string)  [unwired: 3 in]
        n363 = Build Path(base path=w693, name or relative path="t0.txt") -> (appended path=w697:path)
        n364 = Write to Text File(file (use dialog)=w697, text=w695) -> ()  [unwired: 2 in, 3 out]
      }
      event "ESP_+", "ESP_-": Value Change {
        n365 = event-data() -> ()  [unwired: 1 in, 6 out]
        n366 = Negate(x="ESP_delta") -> (-x=w707:dbl)
        n367 = Select(t="ESP_delta", s="ESP_+", f=w707) -> (s? t:f=w705:dbl)
        n368 = Number To Decimal String(number="ESP Axis") -> (decimal integer string=w702:string)  [unwired: 1 in]
        n369 = Number To Fractional String(number=w705) -> (F-format string=w700:string)  [unwired: 3 in]
        n370 = Concatenate Strings("rel:" ("string"), w702, ":" ("string"), w700) -> (w710:string)
        n371 = Enqueue Element(queue=w704, element=w710) -> ()  [unwired: 2 in, 3 out]
      }
      event "ESP_dest": Value Change {
        n372 = event-data() -> ()  [unwired: 1 in, 6 out]
        n373 = local read "ESP_dest"() -> (w714:dbl)
        n374 = local read "ESP_t0"() -> (w713:dbl)
        n375 = call "mm2time.vi"("fs?"=TRUE ("fs[1]/ps[0]"), "Offset (mm)"=w713, "distance (mm)"=w714) -> ("time in fs/ps seconds"=w711:dbl)
        n376 = local write "ESP_dest_t"(w711) -> ()
      }
      event "ESP_dest_t": Value Change {
        n377 = event-data() -> ()  [unwired: 1 in, 1 out]
        n378 = local read "ESP_t0"() -> (w717:dbl)
        n379 = call "time2mm.vi"("fs[1]/ps[0]"=TRUE, "Offset (mm)"=w717, "time"="ESP_dest_t") -> ("position (mm)"=w715:dbl)
        n380 = local write "ESP_dest"(w715) -> ()
      }
    }
  }
  n381 = while {
    tunnel: w13 -> [w727]
    shift-right: [w725] -> _
    shift-left: _ -> [w723]
    shift-right: [w724] -> _
    shift-left: _ -> [w722]
    shift-right: [w720] -> _
    shift-left: 0 -> [w721]
    tunnel: w2 -> [w719]
    stop <- w726 stop-if-true
    # "ESP"
    n382 = Preview Queue Element(queue=w727, timeout in ms (-1)=w721) -> (queue out=w730:refnum<queue>, element=w731:string)  [unwired: 1 in, 2 out]
    n383 = Match Pattern(string=w731, regular expression=":") -> (before substring=w729:string, after substring=w728:string)  [unwired: 1 in, 2 out]
    n384 = case shown="\"idle\", Default" w729 {
      tunnel: w730 -> [_ w742 w760 w794 w795 w802 w807]
      tunnel: w728 -> [_ w747 w767 _ _ _ _]
      tunnel: [_ _ _ _ _ TRUE _] -> w726
      tunnel: [w734 w749 w761 w792 refnum<visa-resource-name> refnum ("VISA resource name out") w799 w806] -> w725
      tunnel: [w733 w750 w759 w791 w797 w800 w805] -> w724
      tunnel: w723 -> [w738 w752 w765 w792 w798 w799 _]
      tunnel: w722 -> [w737 w751 w766 w791 _ w800 _]
      tunnel: [_ _ _ -1 _ _ _] -> w720
      tunnel: w719 -> [_ _ w758 _ _ _ _]
      frame "idle", Default {
        n385 = local read "ESP Axis"() -> (w735:i32)
        n386 = local read "ESP_t0"() -> (w741:dbl)
        n387 = call "Read Actual Position.vi"("error in (no error)"=w737, "Axis (1)"=w735, "VISA resource name"=w738) -> ("error out"=w733:errorcluster, "Position (units)"=w736:dbl, "VISA resource name out"=w734:refnum<visa-resource-name>)  [unwired: 2 in]
        "ESP_pos" <- w736
        n388 = call "mm2time.vi"("fs?"=TRUE, "Offset (mm)"=w741, "distance (mm)"=w736) -> ("time in fs/ps seconds"=→"ESP_delay":dbl)
      }
      frame "rel" {
        n389 = Match Pattern(string=w747, regular expression=":") -> (before substring=w746:string, after substring=w745:string)  [unwired: 1 in, 2 out]
        n390 = Dequeue Element(queue=w742) -> ()  [unwired: 2 in, 4 out]
        n391 = Decimal String To Number(string=w746) -> (number=w744:i32)  [unwired: 2 in, 1 out]
        n392 = Fract/Exp String To Number(string=w745) -> (number=w743:dbl)  [unwired: 3 in, 1 out]
        n393 = call "Move Relative.vi"("error in (no error)"=w751, "Position (0 units)"=w743, "Axis (1)"=w744, "VISA resource name"=w752) -> ("error out"=w750:errorcluster, "VISA resource name out"=w749:refnum<visa-resource-name>)  [unwired: 2 in]
      }
      frame "abs" {
        n394 = Dequeue Element(queue=w760) -> ()  [unwired: 2 in, 4 out]
        n395 = Match Pattern(string=w767, regular expression=":") -> (before substring=w768:string, after substring=w756:string)  [unwired: 1 in, 2 out]
        n396 = Match Pattern(string=w756, regular expression=":") -> (before substring=w755:string, after substring=w754:string)  [unwired: 1 in, 2 out]
        n397 = Decimal String To Number(string=w768) -> (number=w764:i32)  [unwired: 2 in, 1 out]
        n398 = Fract/Exp String To Number(string=w755) -> (number=w753:dbl)  [unwired: 3 in, 1 out]
        n399 = call "Move Absolute.vi"("error in (no error)"=w766, "Position (0 units)"=w753, "Axis (1)"=w764, "VISA resource name"=w765) -> ("error out"=w762:errorcluster, "VISA resource name out"=w763:refnum<visa-resource-name>)  [unwired: 2 in]
        n400 = case shown="\"wait\"" w754 {
          tunnel: w764 -> [_ w776]
          tunnel: w763 -> [w771 w781]
          tunnel: w762 -> [w770 w780]
          tunnel: [w771 w773] -> w761
          tunnel: [w770 w779] -> w759
          tunnel: w758 -> [_ w778]
          frame "", Default {
          }
          frame "wait" {
            n401 = while {
              tunnel: w776 -> [w790]
              shift-right: [w787] -> w775
              shift-left: w781 -> [w789]
              shift-right: [w786] -> w774
              shift-left: w780 -> [w788]
              stop <- w785 stop-if-true
              n402 = call "Get Axis Motion Status.vi"("error in (no error)"=w788, "Axis (1)"=w790, "VISA resource name"=w789) -> ("error out"=w786:errorcluster, "Motion Done"=w785:bool, "VISA resource name out"=w787:refnum<visa-resource-name>)  [unwired: 2 in]
            }
            n403 = flat-sequence {
              tunnel: w775 -> [w784]
              tunnel: w774 -> [w783]
              tunnel: [w784] -> w773
              tunnel: [w783] -> w772
              frame #0 {
                n404 = Wait (ms)(milliseconds to wait=u32 1000) -> ()  [unwired: 1 out]
              }
            }
            n405 = Enqueue Element(queue=w778, element="done", error in (no error)=w772) -> (error out=w779:errorcluster)  [unwired: 1 in, 2 out]
          }
        }
      }
      frame "suspend" {
        n406 = Dequeue Element(queue=w794) -> ()  [unwired: 2 in, 4 out]
      }
      frame "release" {
        n407 = Dequeue Element(queue=w795) -> ()  [unwired: 2 in, 4 out]
        n408 = call "Close.vi"("VISA resource name"=w798) -> ("error out"=w797:errorcluster)  [unwired: 10 in]
      }
      frame "close" {
        n409 = Release Queue(queue=w802) -> ()  [unwired: 2 in, 3 out]
      }
      frame "init" {
        n410 = Dequeue Element(queue=w807) -> ()  [unwired: 2 in, 4 out]
        n411 = flat-sequence {
          tunnel: [w810] -> w804
          tunnel: [w809] -> w803
          tunnel: [w814] -> w805
          tunnel: [w815] -> w806
          tunnel: w804 -> [w815]
          tunnel: w803 -> [w814]
          frame #0 {
            n412 = local write "ESP_con?"(FALSE ("ESP_con?")) -> ()
          }
          frame #1 {
            n413 = call "Initialize.vi"("VISA resource name"="ESP301 VISA", "Serial Link (RS232)"=enum16{"RS232", "USB"}."USB") -> ("VISA resource name out"=w810:refnum<visa-resource-name>, "error out"=w809:errorcluster)  [unwired: 7 in]
          }
          frame #2 {
            n414 = local write "ESP_con?"(TRUE ("ESP_con?")) -> ()
          }
        }
      }
    }
    "error out" <- w724
  }
  n415 = while {
    tunnel: w3 -> [w824]
    shift-right: [w822] -> _
    shift-left: _ -> [w820]
    shift-right: [w821] -> _
    shift-left: _ -> [w819]
    shift-right: [w817] -> _
    shift-left: 0 -> [w818]
    tunnel: w2 -> [w816]
    stop <- w823 stop-if-true
    # "manip"
    n416 = Preview Queue Element(queue=w824, timeout in ms (-1)=w818) -> (queue out=w827:refnum<queue>, element=w828:string)  [unwired: 1 in, 2 out]
    n417 = Match Pattern(string=w828, regular expression=":") -> (before substring=w826:string, after substring=w825:string)  [unwired: 1 in, 2 out]
    n418 = case shown="\"idle\", Default" w826 {
      tunnel: w827 -> [_ w840 w867 w894 w898 w907 w912]
      tunnel: w825 -> [_ _ w854 _ _ _ _]
      tunnel: [_ _ _ _ _ TRUE _] -> w823
      tunnel: [w834 w842 w846 w896 refnum<k5> refnum ("gateway_connection out") w905 w911] -> w822
      tunnel: [w833 w841 w848 w895 w900 w904 w910] -> w821
      tunnel: w820 -> [w836 w844 w870 w896 w902 w905 _]
      tunnel: w819 -> [w835 w843 w869 w895 _ w904 _]
      tunnel: [_ _ _ -1 _ _ _] -> w817
      tunnel: w816 -> [_ _ w845 _ _ _ _]
      frame "idle", Default {
        n419 = call "sp_manip_get_axis_status.vi"("error in"=w835, "gateway_connection"=w836) -> ("error out"=w833:errorcluster, "axis_out"=w832:T7, "gateway_connection out"=w834:refnum<k5>)  [unwired: 5 in, 2 out]
        n420 = for {
          tunnel: w832 -> [w839] mode=indexing
          tunnel: [w838] -> w831 mode=indexing
          tunnel: [w837] -> w830 mode=indexing
          n421 = Unbundle By Name(w839) -> ("Axis_Position"=w838:dbl, "moving"=w837:bool)
        }
        "moving?" <- w830
        n422 = local write "pos"(w831) -> ()
      }
      frame "stop" {
        n423 = Dequeue Element(queue=w840) -> ()  [unwired: 2 in, 4 out]
        n424 = call "sp_manip_abort.vi"("error in"=w843, "gateway_connection"=w844) -> ("error out"=w841:errorcluster, "gateway_connection out"=w842:refnum<k5>)  [unwired: 6 in, 2 out]
      }
      frame "relative" {
        n425 = Dequeue Element(queue=w867) -> ()  [unwired: 2 in, 4 out]
        n426 = Match Pattern(string=w854, regular expression=":") -> (before substring=w853:string, after substring=w852:string)  [unwired: 1 in, 2 out]
        n427 = Equal?(x=w852, y="wait") -> (x = y?=w850:bool)
        n428 = call "sp_manip_get_axis_status.vi"("error in"=w869, "gateway_connection"=w870) -> ("error out"=w872:errorcluster, "axis_out"=w859:T7, "gateway_connection out"=w871:refnum<k5>)  [unwired: 5 in, 2 out]
        n429 = Scan From String(format string="%g_%g_%g_%g_%g_%g", input string=w853) -> (output 1=w866:dbl, output 2=w865:dbl, output 3=w864:dbl, output 4=w863:dbl, output 5=w862:dbl, output 6=w861:dbl)  [unwired: 8 in, 3 out]
        n430 = for {
          tunnel: w859 -> [w893] mode=indexing
          tunnel: [w892] -> w857 mode=indexing
          tunnel: [w891] -> w858 mode=indexing
          n431 = Unbundle By Name(w893) -> ("Axis_Name"=w892:string, "Axis_Position"=w891:dbl)
        }
        n432 = Build Array(w866, w865, w864, w863, w862, w861) -> (w860:dbl[])
        n433 = Add(x=w858, y=w860) -> (x+y=w856:dbl[])
        n434 = call "sp_manip_start_move.vi"("error in"=w872, "target positions"=w856, "axis names"=w857, "gateway_connection"=w871) -> ("error out"=w849:errorcluster, "gateway_connection out"=w847:refnum<k5>)  [unwired: 4 in, 2 out]
        n435 = case shown="True" w850 {
          tunnel: w849 -> [w873 w880]
          tunnel: [w873 w876] -> w848
          tunnel: w847 -> [w874 w881]
          tunnel: [w874 w879] -> w846
          tunnel: w845 -> [_ w875]
          frame False {
          }
          frame True {
            n436 = while {
              tunnel: w881 -> [w885]
              tunnel: w880 -> [w884]
              tunnel: [w883] -> w879
              tunnel: [w882] -> w877
              stop <- w886 continue-if-true
              n437 = call "sp_manip_get_axis_status.vi"("error in"=w884, "gateway_connection"=w885) -> ("error out"=w882:errorcluster, "axis_out"=w888:T7, "gateway_connection out"=w883:refnum<k5>)  [unwired: 5 in, 2 out]
              n438 = for {
                tunnel: w888 -> [w890] mode=indexing
                tunnel: [w889] -> w887 mode=indexing
                n439 = Unbundle By Name(w890) -> ("moving"=w889:bool)
              }
              n440 = Or Array Elements(Boolean array=w887) -> (logical OR=w886:bool)
            }
            n441 = Enqueue Element(queue=w875, element="done", error in (no error)=w877) -> (error out=w876:errorcluster)  [unwired: 1 in, 2 out]
          }
        }
      }
      frame "suspend" {
        n442 = Dequeue Element(queue=w894) -> ()  [unwired: 2 in, 4 out]
      }
      frame "release" {
        n443 = Dequeue Element(queue=w898) -> ()  [unwired: 2 in, 4 out]
        n444 = call "sp_manip_disconnect.vi"("gateway_connection"=w902) -> ("error out"=w901:errorcluster, "gateway_connection_out"=w903:refnum<k5>)  [unwired: 7 in, 2 out]
        n445 = call "tcp_gateway_close_connection.vi"("error in"=w901, "server_connection"=w903) -> ("error out"=w900:errorcluster)  [unwired: 5 in]
      }
      frame "close" {
        n446 = Release Queue(queue=w907) -> ()  [unwired: 2 in, 3 out]
      }
      frame "init" {
        n447 = Dequeue Element(queue=w912) -> ()  [unwired: 2 in, 4 out]
        n448 = flat-sequence {
          tunnel: [w915] -> w909
          tunnel: [w914] -> w908
          tunnel: [w925] -> w910
          tunnel: [w926] -> w911
          tunnel: w909 -> [w926]
          tunnel: w908 -> [w925]
          frame #0 {
            n449 = local write "manip_con?"(FALSE ("manip_con?")) -> ()
          }
          frame #1 {
            n450 = call "tcp_gateway_open_connection.vi"() -> ("gateway_connection"=w918:refnum<k5>, "error out"=w917:errorcluster)  [unwired: 5 in, 3 out]
            n451 = call "sp_manip_connect.vi"("error in"=w917, "gateway_connection"=w918) -> ("error out"=w914:errorcluster, "axis_out"=w916:T7, "gateway_connection out"=w915:refnum<k5>)  [unwired: 5 in, 2 out]
            n452 = for {
              tunnel: w916 -> [w923] mode=indexing
              tunnel: [w922] -> w919 mode=indexing
              tunnel: [w921] -> w920 mode=indexing
              n453 = Unbundle By Name(w923) -> ("Axis_Name"=w922:string, "Axis_Position"=w921:dbl)
            }
            "axis" <- w919
            "pos" <- w920
            n454 = local write "dest"(w920) -> ()
          }
          frame #2 {
            n455 = local write "manip_con?"(TRUE ("manip_con?")) -> ()
          }
        }
      }
    }
    "error out 2" <- w821
  }
  n456 = while {
    tunnel: w24 -> [w937]
    shift-right: [w934] -> _
    shift-left: 0 -> [w935]
    shift-right: [w933] -> _
    shift-left: _ -> [w932]
    shift-right: [w931] -> _
    shift-left: _ -> [w930]
    shift-right: [w929] -> _
    shift-left: u32 0 ("pHandle") -> [w928]
    tunnel: string[] ["Kinetic Energy", "Pass Energy", "Coil Current", "Work Function", "Detector Voltage", "Screen Voltage", "Conversion Voltage", "Focus Displacement 1", "Focus Displacement 2"] -> [w927]
    stop <- w936 stop-if-true
    # "phoib"
    n457 = Preview Queue Element(queue=w937, timeout in ms (-1)=w935) -> (queue out=w940:refnum<queue>, element=w941:string)  [unwired: 1 in, 2 out]
    n458 = Match Pattern(string=w941, regular expression=":") -> (before substring=w939:string, after substring=w938:string)  [unwired: 1 in, 2 out]
    n459 = case shown="\"standby\"" w939 {
      tunnel: w940 -> [_ w994 w1010 w1026 w1040 w1044 w1050]
      tunnel: w938 -> [_ _ _ _ _ _ _]
      tunnel: [_ _ _ _ TRUE _ _] -> w936
      tunnel: [_ _ _ _ _ -1 _] -> w934
      tunnel: [w951 w996 w1013 w1024 w1038 w1043 w1047] -> w933
      tunnel: w932 -> [w962 w985 w1015 w1025 w1038 w1043 _]
      tunnel: [w950 w995 w1012 w1023 w1036 w1041 w1046] -> w931
      tunnel: w930 -> [w960 w984 w1014 _ w1036 w1041 _]
      tunnel: [w948 w982 w1011 w1022 w1037 w1042 w1049] -> w929
      tunnel: w928 -> [w948 w982 w1011 w1021 w1037 w1042 _]
      tunnel: w927 -> [w949 w975 _ _ _ _ _]
      frame "idle", Default {
        n460 = call "SL2_AD_DLL_Phoibos_GetDeviceState.vi"("dll_path"=w962, "pHandle_in"=w948, "dev_type"=DEF_dev_type."devA (analyzer)", "error in"=w960) -> ("path out"=w947:path, "state"=→"state":T3, "error out"=w946:errorcluster)  [unwired: 2 in]
        n461 = for {
          tunnel: w948 -> [w969]
          tunnel: w949 -> [w967] mode=indexing
          tunnel: [w966] -> w959 mode=indexing
          tunnel: [w965] -> w951
          shift-right: [w964] -> w950
          shift-left: w946 -> [w968]
          tunnel: w947 -> [w963]
          n462 = call "SL2_AD_DLL_Phoibos_GetVoltage.vi"("error in"=w968, "voltage_name"=w967, "pHandle"=w969, "dll path in"=w963) -> ("error out"=w964:errorcluster, "value"=w966:dbl, "dll path out"=w965:path)  [unwired: 3 in]
        }
        n463 = Index Array(array=w959) -> (element #1=→"phoib_I_1":dbl, element #2=→"phoib_I_2":dbl, element #3=→"phoib_I_3":dbl, element #4=→"phoib_I_4":dbl, element #5=→"phoib_I_5":dbl, element #6=→"phoib_I_6":dbl, element #7=→"phoib_I_7":dbl, element #8=→"phoib_I_8":dbl, element #9=→"phoib_I_9":dbl)  [unwired: 9 in]
      }
      frame "set" {
        n464 = Dequeue Element(queue=w994) -> ()  [unwired: 2 in, 4 out]
        n465 = Multiply(x="VoltageRange", y=13) -> (x*y=w991:i32)
        n466 = Add(x="Mode", y=w991) -> (x+y=w988:i32)
        n467 = Index Array(array=u32[] [251749632, 251749633, 251749634, 251749635, 251749636, 251749637, 251749638, 251749639, 251749640, 251749641, 251749642, 251749643, 251749644, 251749645, 251749646, 251749647, 251749648, 251749649, 251749650, 251749651, 251749652, 251749653, 251749654, 251749655, 251749656, 251749657, 251749658, 251749659, 251749660, 251749661, 251749662, 251749663, 251749664, 251749665, 251749666, 251749667, 251749668, 251749669, 251749670, 251749671, 251749672, 251749673, 251749674, 251749675, 251749676, 251749677, 251749678, 251749679, 251749680, 251749681, 251749682, 251749683, 251749684, 251749685, 251749686, 251749687, 251749688, 251749689, 251749690, 251749691, 251749692, 251749693, 251749694, 251749695, 251749696] ("modeIDs"), index=w988) -> (element=w986:u32)
        n468 = Build Array("phoib_I_1s", "phoib_I_2s", "phoib_I_3s", "phoib_I_4s", "phoib_I_5s", "phoib_I_6s", "phoib_I_7s", "phoib_I_8s", "phoib_I_9s") -> (w974:dbl[])
        n469 = call "SL2_AD_DLL_Phoibos_SetDeviceMode.vi"("pHandle"=w982, "error in"=w984, "value"=w986, "dev_type"=DEF_dev_type."devA (analyzer)", "dll path in"=w985) -> ("error out"=w973:errorcluster, "dll path out"=w983:path)  [unwired: 4 in]
        n470 = for {
          tunnel: w982 -> [w1002]
          shift-right: [w1009] -> w996
          shift-left: w983 -> [w1006]
          tunnel: w975 -> [w1001] mode=indexing
          tunnel: w974 -> [w1000] mode=indexing
          shift-right: [w1008] -> w995
          shift-left: w973 -> [w1004]
          n471 = call "SL2_AD_DLL_Phoibos_GetVoltageRange.vi"("error in"=w1004, "voltage_name"=w1001, "pHandle"=w1002, "dll path in"=w1006) -> ("error out"=w1003:errorcluster, "min"=w998:dbl, "max"=w999:dbl, "dll path out"=w1005:path)  [unwired: 2 in]
          n472 = In Range and Coerce(upper limit=w999, x=w1000, lower limit=w998) -> (coerced(x)=w997:dbl)  [unwired: 1 out]
          n473 = call "SL2_AD_DLL_Phoibos_SetVoltage.vi"("commit"=TRUE, "pHandle"=w1002, "error in"=w1003, "value"=w997, "voltageName"=w1001, "dll path in"=w1005) -> ("error out"=w1008:errorcluster, "dll path out"=w1009:path)  [unwired: 3 in]
        }
      }
      frame "standby" {
        w1016 = T3 0 items=["Off"=-1, "Standby"=0, "On"=1] ("state")
        n474 = Dequeue Element(queue=w1010) -> ()  [unwired: 2 in, 4 out]
        n475 = call "SL2_AD_DLL_Phoibos_SetDeviceState.vi"("pHandle_in"=w1011, "error in"=w1014, "state"=w1016, "dev_type"=DEF_dev_type."devA (analyzer)", "dll_path"=w1015) -> ("error out"=w1012:errorcluster, "path out"=w1013:path)  [unwired: 2 in]
      }
      frame "release" {
        n476 = Dequeue Element(queue=w1026) -> ()  [unwired: 2 in, 4 out]
        n477 = flat-sequence {
          tunnel: w1025 -> [w1027]
          tunnel: w1021 -> [w1028]
          tunnel: [w1031] -> w1020
          tunnel: [w1030] -> w1019
          tunnel: [u32 0] -> w1018
          tunnel: [w1033] -> w1022
          tunnel: [w1034] -> w1023
          tunnel: [w1035] -> w1024
          tunnel: w1020 -> [w1035]
          tunnel: w1019 -> [w1034]
          tunnel: w1018 -> [w1033]
          frame #0 {
            n478 = call "SL2_AD_DLL_Phoibos_Shutdown.vi"("pHandle"=w1028, "dll path in"=w1027) -> ("error out"=w1030:errorcluster, "dll path out"=w1031:path)  [unwired: 4 in]
          }
          frame #1 {
            n479 = local write "phoib_con?"(FALSE ("phoib_con?")) -> ()
          }
        }
      }
      frame "close" {
        n480 = Release Queue(queue=w1040) -> ()  [unwired: 2 in, 3 out]
      }
      frame "suspend" {
        n481 = Dequeue Element(queue=w1044) -> ()  [unwired: 2 in, 4 out]
      }
      frame "init" {
        n482 = Dequeue Element(queue=w1050) -> ()  [unwired: 2 in, 4 out]
        n483 = flat-sequence {
          tunnel: [w1057] -> w1048
          tunnel: [w1053] -> w1047
          tunnel: [w1052] -> w1046
          tunnel: [w1065] -> w1049
          tunnel: w1048 -> [w1065]
          frame #0 {
            n484 = local write "phoib_con?"(FALSE ("phoib_con?")) -> ()
          }
          frame #1 {
            w1056 = DEF_dev_type."devA (analyzer)" ("dev_type")
            n485 = call "GetSL2AD_VI_dllPath.vi"() -> ("error"=w1060:errorcluster, "Path"=w1061:path)  [unwired: 9 in, 1 out]
            n486 = call "SL2_AD_DLL_List_Devices.vi"("error in"=w1060, "dev_type"=w1056, "dll path in"=w1061) -> ("error out"=w1054:errorcluster, "devices"=w1063:string[], "dll path out"=w1055:path)  [unwired: 2 in]
            n487 = Index Array(array=w1063) -> (element=w1062:string)  [unwired: 1 in]
            n488 = call "SL2_AD_DLL_Phoibos_Initialize.vi"("error in"=w1054, "analyzerId"=w1062, "dll_path"=w1055) -> ("error out"=w1058:errorcluster, "pHandle"=w1057:u32, "path out"=w1059:path)  [unwired: 2 in]
            n489 = call "SL2_AD_DLL_Phoibos_ListDeviceModes.vi"("dll path in"=w1059, "dev_type"=w1056, "pHandle"=w1057, "error in"=w1058) -> ("dll path out"=w1053:path, "error out"=w1052:errorcluster)  [unwired: 1 in, 2 out]
          }
          frame #2 {
            n490 = local write "phoib_con?"(TRUE ("phoib_con?")) -> ()
          }
        }
      }
    }
    "phoib_error" <- w931
  }
